vi "MainScan.vi"() -> ()   [LabVIEW 2012]
uses:
  <userlib>/Circular Buffer/Controls/Circular Buffer Operations.ctl
  <vilib>/DAQmx/write.llb/DAQmx Write (Digital Bool 1Line 1Point).vi
  <vilib>/DAQmx/write.llb/DAQmx Write (Analog 1D DBL NChan 1Samp).vi
  <vilib>/DAQmx/read.llb/DAQmx Read (Analog 1D DBL 1Chan NSamp).vi
  <vilib>/DAQmx/write.llb/DAQmx Write (Analog DBL 1Chan 1Samp).vi
  <vilib>/DAQmx/write.llb/DAQmx Write (Analog 2D DBL NChan NSamp).vi
  <vilib>/DAQmx/read.llb/DAQmx Read (Analog 1D Wfm NChan NSamp).vi
  <vilib>/DAQmx/create/channels.llb/DAQmx Create Channel (DO-Digital Output).vi
  <vilib>/DAQmx/create/channels.llb/DAQmx Create Channel (AO-Voltage-Basic).vi
  <vilib>/DAQmx/create/channels.llb/DAQmx Create Channel (AI-Voltage-Basic).vi
  <vilib>/DAQmx/configure/timing.llb/DAQmx Timing (Sample Clock).vi
  <vilib>/DAQmx/miscellaneous.llb/DAQmx Fill In Error Info.vi
  <vilib>/DAQmx/create/channels.llb/DAQmx Create Channel (CO-Pulse Generation-Frequency).vi
  <vilib>/DAQmx/configure/timing.llb/DAQmx Timing (Implicit).vi
  <vilib>/Analysis/baseanly.llb/Mean (DBL).vi
  <vilib>/DAQmx/configure/trigger.llb/DAQmx Start Trigger (Digital Edge).vi
  <userlib>/Circular Buffer/Instance VIs/Circular Buffer(2D Wfm).vi
  <vilib>/measure/madcrms.llb/Basic Averaged DC-RMS for N Chan.vi
  <resource>/objmgr/daqmx.rc
  <userlib>/Circular Buffer/Circular Buffer.lvlib
  <vilib>/Analysis/NI_AALBase.lvlib
  <vilib>/measure/NI_MAPro.lvlib
panel:
  in  "z-Position":dbl min=0.0 max=10.0
  in  "Schritte":dbl=20.0 min=0.0 step=1.0 format="%#.0f"
  out "Duration (m.s)":string
  in  "Piezo Stage":bool
  in  "maximum":dbl=1.0
  in  "minimum":dbl=-10.0
  out "Sensitivity":string
  out "Phase":string
  out "Lock-in":bool
  in  "green PMT-gain":dbl=5.0
  in  "red PMT-gain":dbl=9.5
  in  "NA 2":dbl=1.3 min=0.0
  in  "Magn":dbl=40.0
  in  "Magn":dbl=100.0
  in  "Buffer Size":i32(ring)=750 items=["1000x"=1000, "750x"=750, "500x"=500, "250x"=250, "150x"=150, "100x"=100, "50x"=50, "20x"=20]
  out "Buffer":dbl(slide) scale=0.0..1.0
  out "Mira Power (mW)":dbl format="%.2f"
  in  "Scanrate (pixels/s)":i32(ring)=50 items=["250 kHz"=250000, "200 kHz"=200000, "100 kHz"=100000, "50 kHz"=50000, "25 kHz"=25000, "20 kHz"=20000, "10 kHz"=10000, "5 kHz"=5000, "2 kHz"=2000, "1 kHz"=1000, "500 Hz"=500, "200 Hz"=200, "100 Hz"=100, "50 Hz"=50, "20 Hz"=20, "10 Hz"=10, "5 Hz"=5, "2 Hz"=2, "1 Hz"=1]
  out "Optimal":string
  out "Pixel [nm]":dbl format="%#.0f"
  in  "Pulse width fs":dbl=270.0 min=0.0
  in  "Power mW nosync":dbl=1.0 min=0.0
  in  "Power mW sync":dbl=1.0 min=0.0
  in  "Power mA":dbl=1.0 min=0.0
  in  "HWP":dbl=20.0 min=0.0 step=2.5
  in  "NA":dbl=1.2 min=0.0
  in  "Fire":bool
  in  "Pulse repetition rate":dbl(ring)=250000.0 items=["0.5 Hz"=0.5, "1 Hz"=1.0, "2 Hz"=2.0, "5 Hz"=5.0, "10 Hz"=10.0, "20 Hz"=20.0, "50 Hz"=50.0, "100 Hz"=100.0, "200 Hz"=200.0, "500 Hz"=500.0, "1 kHz"=1000.0, "2 kHz"=2000.0, "5 kHz"=5000.0, "10 kHz"=10000.0, "20 kHz"=20000.0, "50 kHz"=50000.0, "100 kHz"=100000.0, "200 kHz"=200000.0, "250 kHz"=250000.0]
  in  "Number of shots":i32(ring)=1 items=["Single"=1, "Double"=2, "5"=5, "10"=10, "20"=20, "50"=50, "100"=100, "200"=200, "500"=500, "1000"=1000, "2000"=2000, "5000"=5000, "10000"=10000, "20000"=20000, "50000"=50000, "100000"=100000, "200000"=200000, "500000"=500000, "Continuos"=0]
  in  "Swap Memory":bool
  out "Memory":dbl[][](graph)
  out "System":bool
  in  "black point":bool
  in  "Magnification":dbl=60.0
  in  "Go home":bool
  in  "Go to white point":bool
  in  "Maximum val":dbl max=100.0 format="%#_4f"
  in  "Minimum val":dbl min=-200.0 step=0.25 format="%#_4f"
  in  "Z-Stacking":bool
  in  "Schrittweite":dbl=1.0 min=0.0
  in  "Minimum":dbl(slide) min=-200.0 max=10.0 step=0.25 scale=-100.0..100.0
  in  "Maximum":dbl(slide)=0.30612244897959184 min=-10.0 max=100.0 scale=-100.0..100.0
  out "path":path
  in  "File identifier":string="unnamed_file"
  in  "Bild speichern ...":bool
  out "Grösse manuell":dbl=22.400000000000002
  in  "Scan":bool
  in  "y-Offset":dbl min=-636.16 max=636.16 format="%#.2f"
  in  "x-Offset":dbl min=-636.16 max=636.16 format="%#.2f"
  in  "Grösse":dbl(ring)=0.04 items=["1x1 µm"=0.005, "2x2 µm"=0.01, "4x4 µm"=0.02, "9x9 µm"=0.04, "18x18 µm"=0.08, "36x36 µm"=0.16, "72x72 µm"=0.32, "143x143 µm"=0.64]
  out "Image":dbl[][](graph)
  in  "Auflösung":i32(ring) items=["512x512"=512, "256x256"=256, "128x128"=128, "64x64"=64, "32x32"=32, "16x16"=16, "8x8"=8, "4x4"=4, "2x2"=2, "1x1"=1, "Optimal"=0]
  # "Auslesebereich"
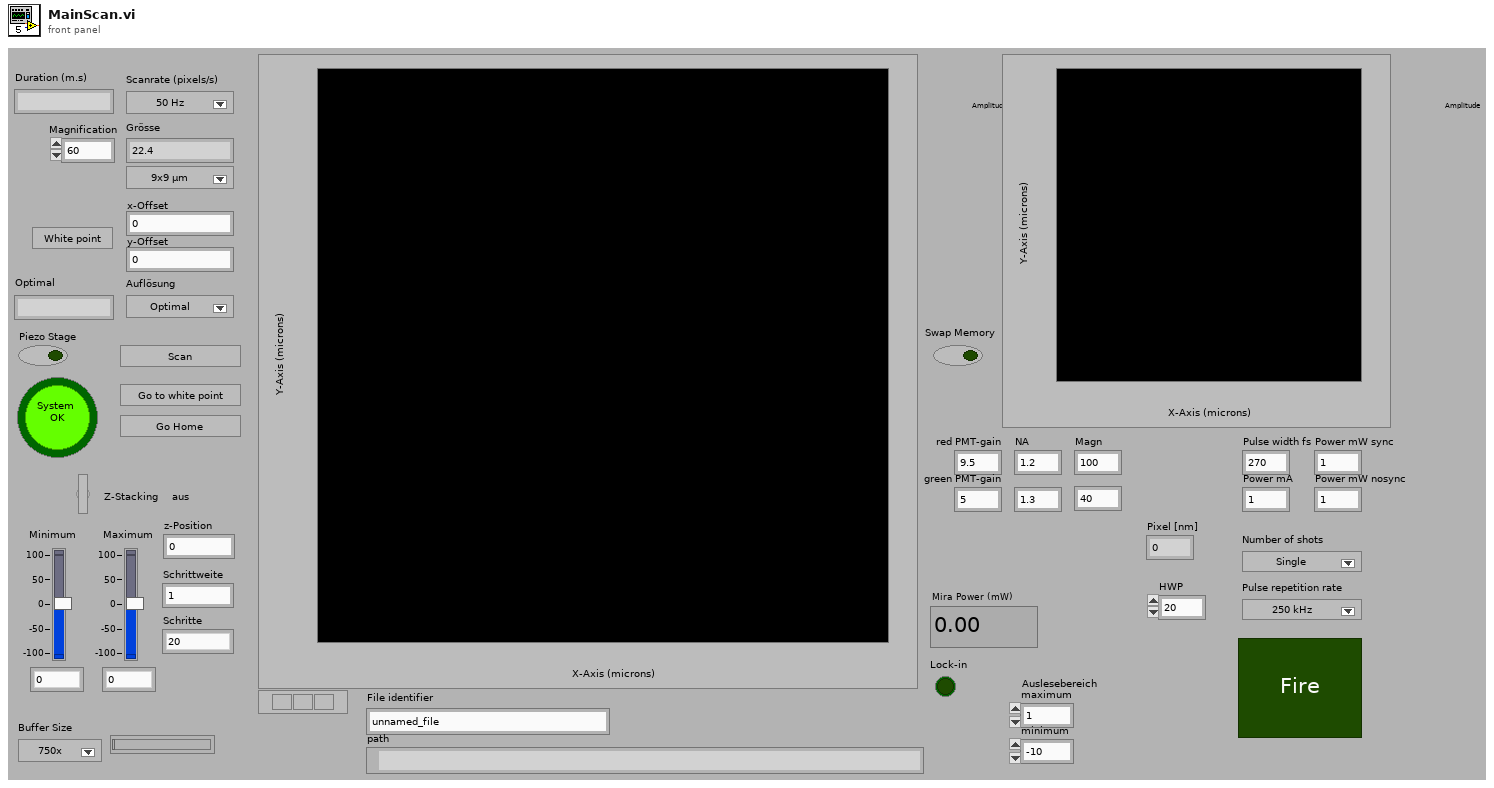
[diagram p1: front panel]
types:
  T1 = typedef "Circular Buffer.lvlib/Circular Buffer Operations.ctl" = enum16{"Initialize", "Get Backlog", "Write", "Read (continuous)", "Read (most recent)"}
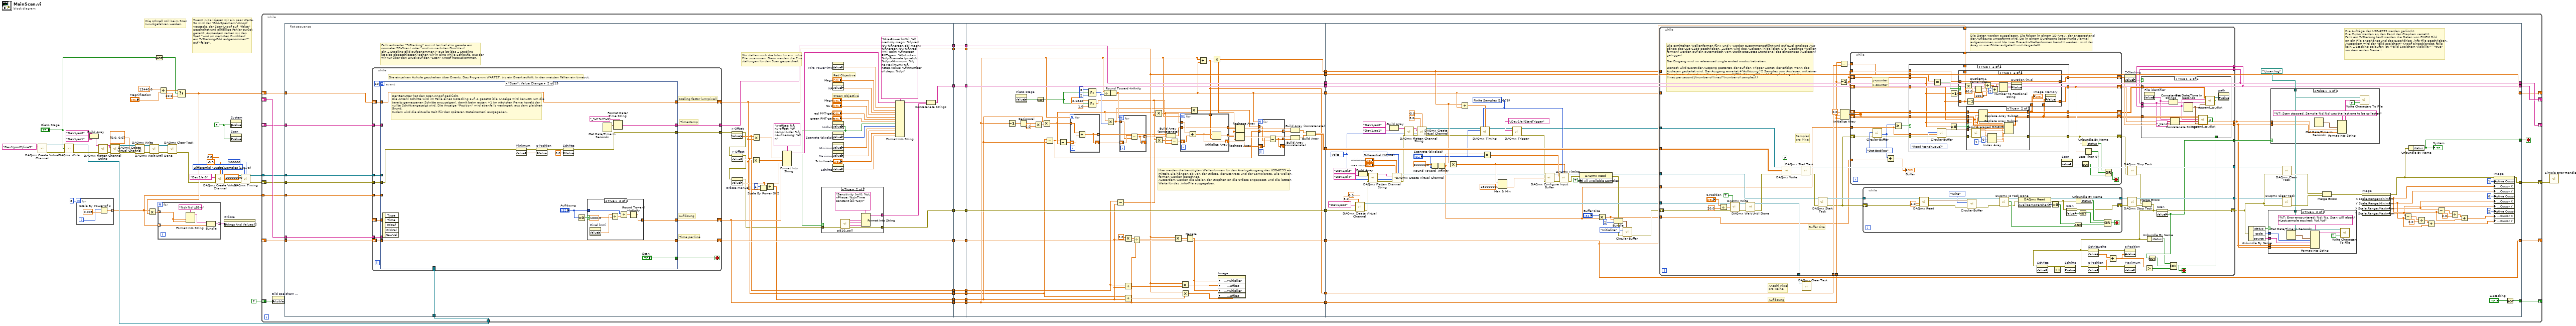
[diagram p0: block diagram]
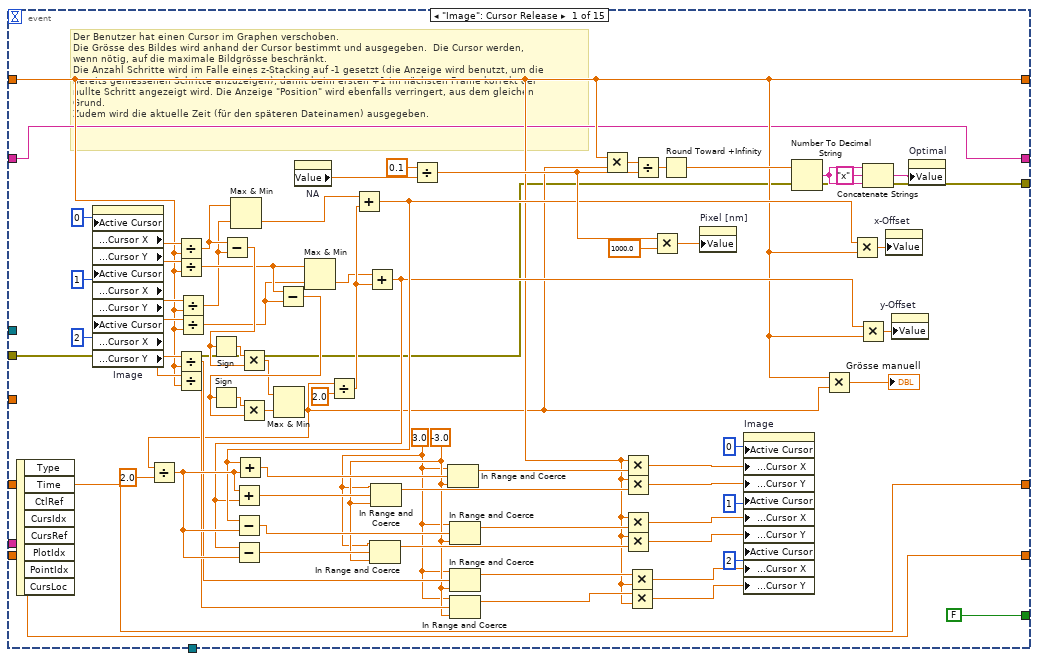
[diagram p2: hidden frame]
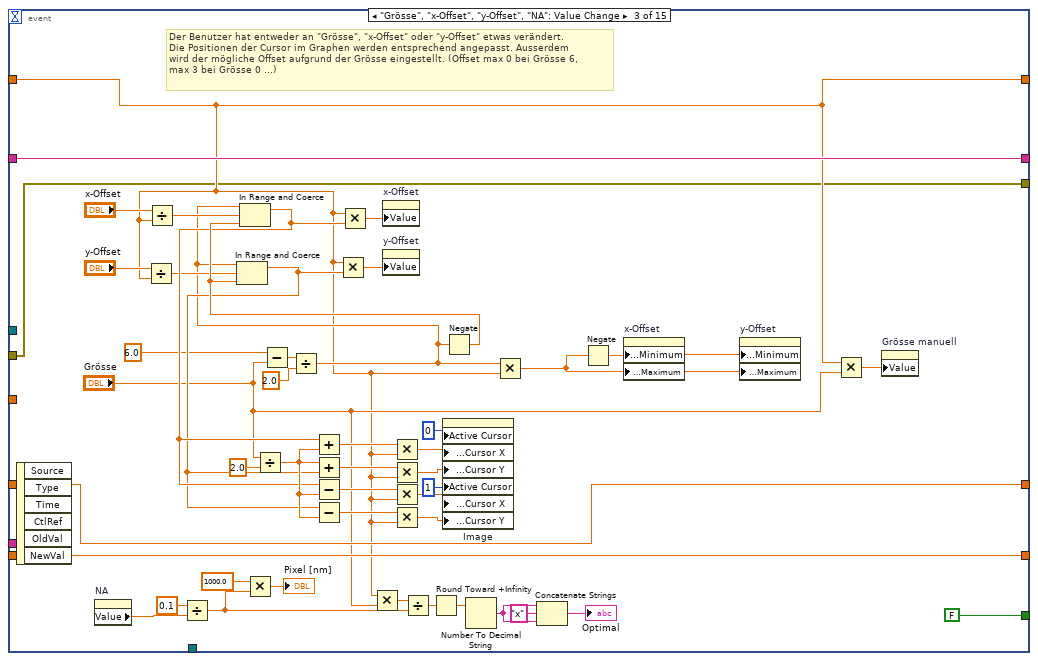
[diagram p4: hidden frame]
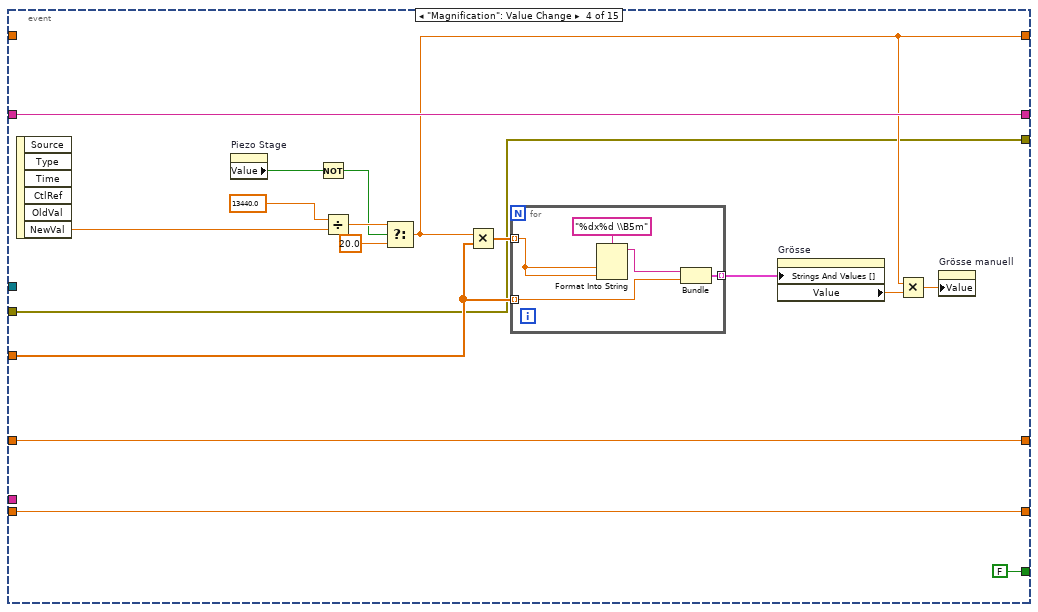
[diagram p5: hidden frame]
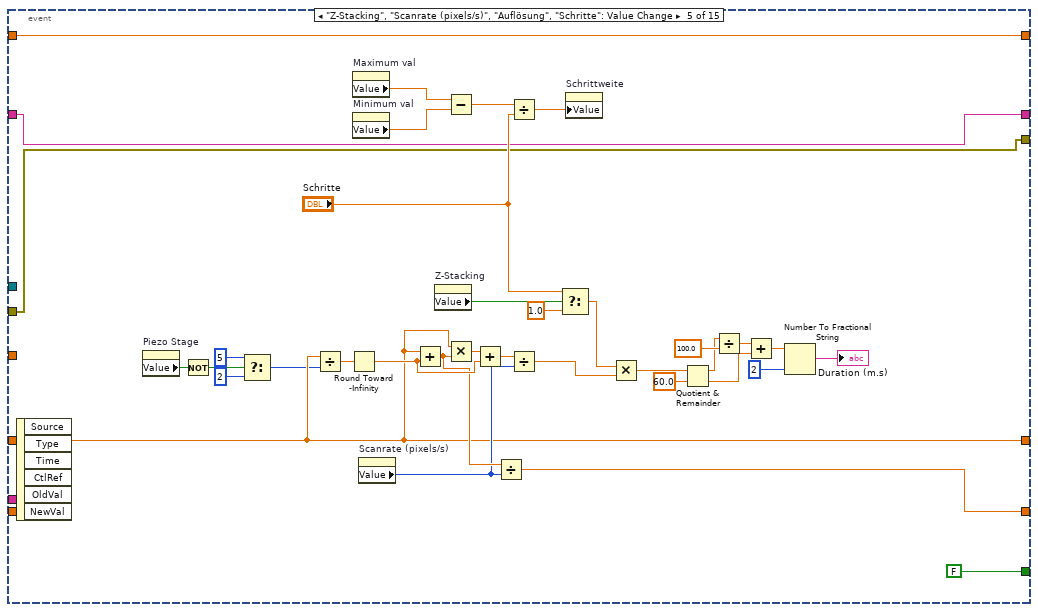
[diagram p6: hidden frame]
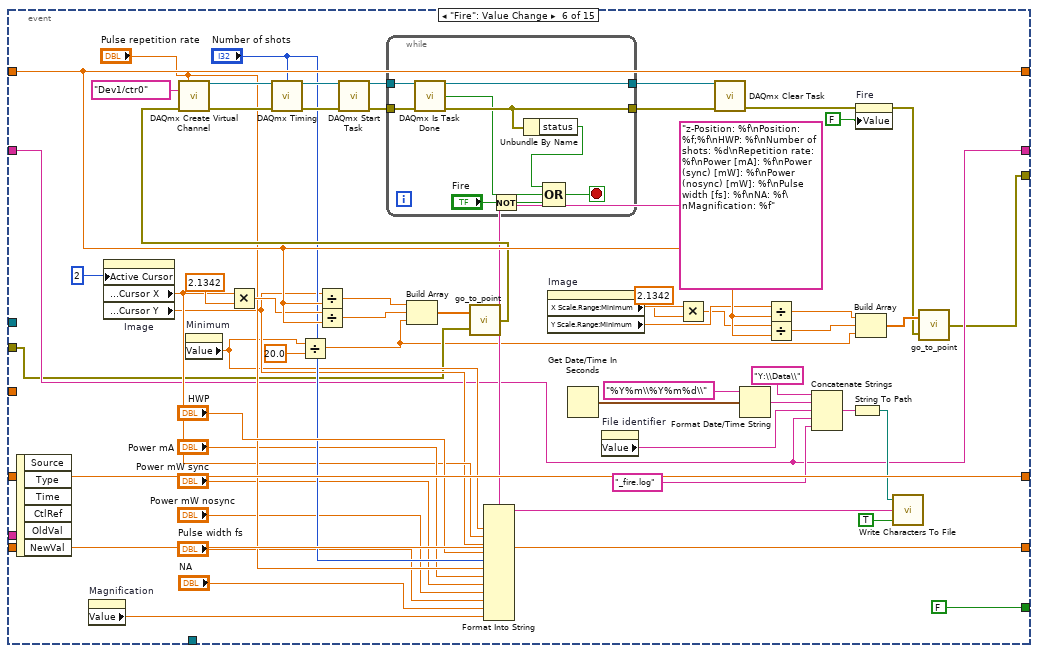
[diagram p7: hidden frame]
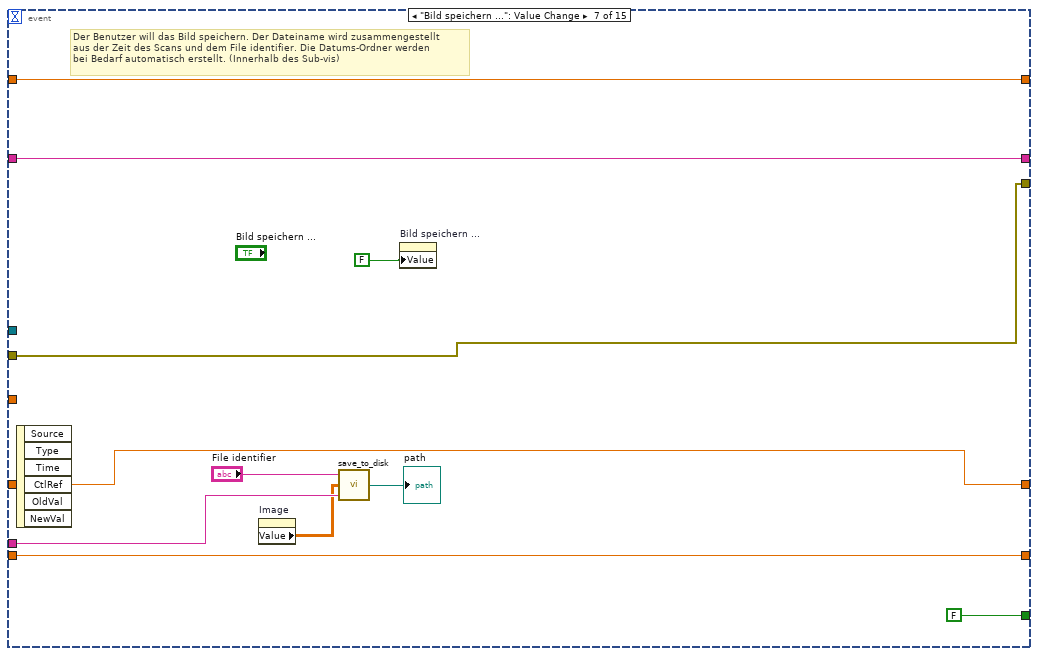
[diagram p8: hidden frame]
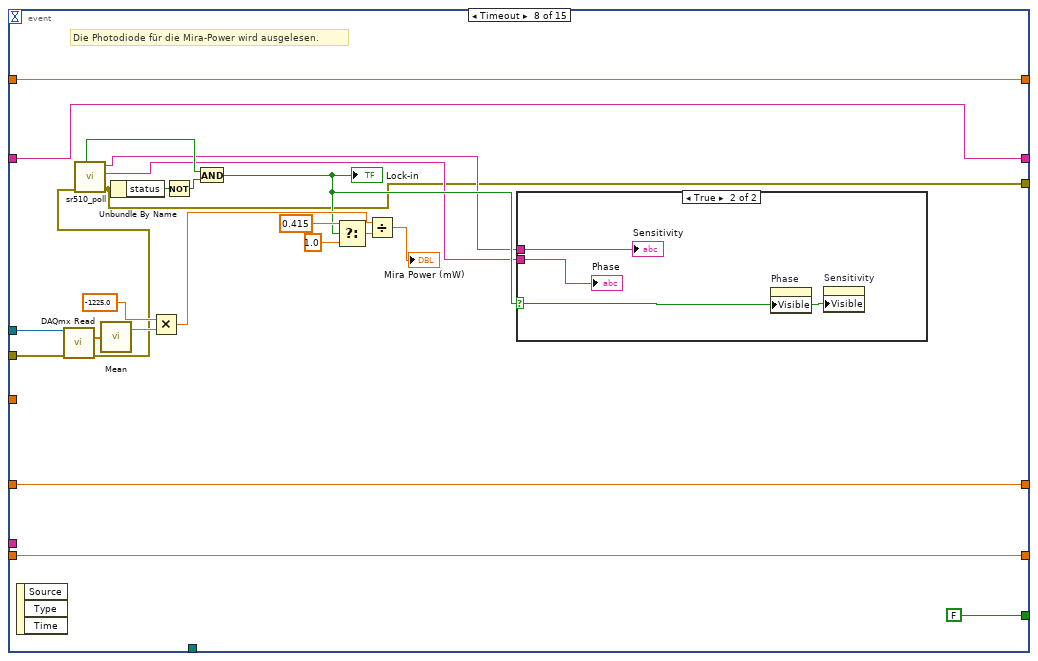
[diagram p9: hidden frame]
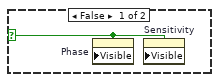
[diagram p10: hidden frame]
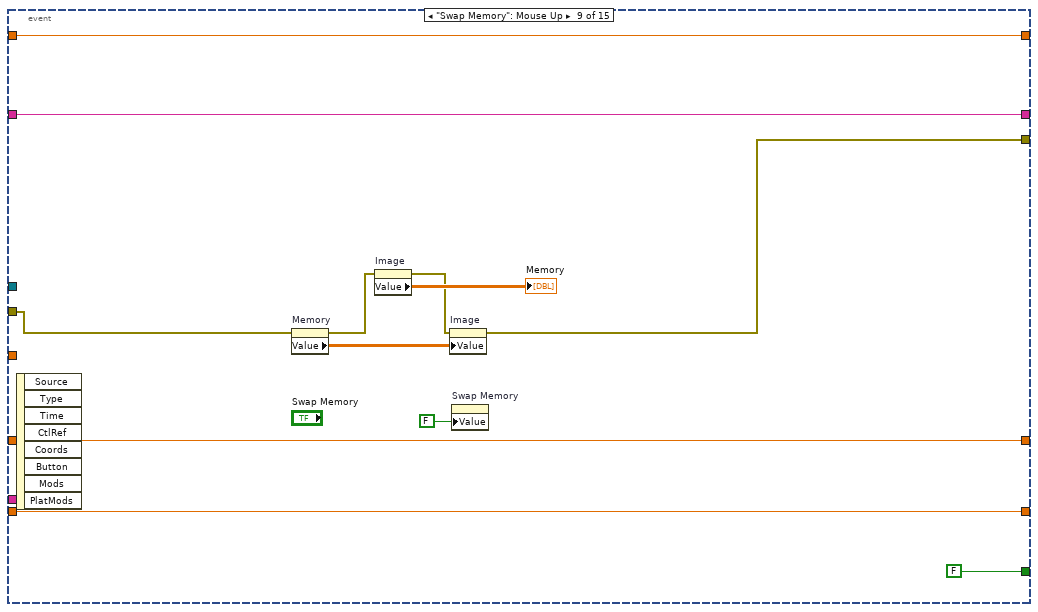
[diagram p11: hidden frame]
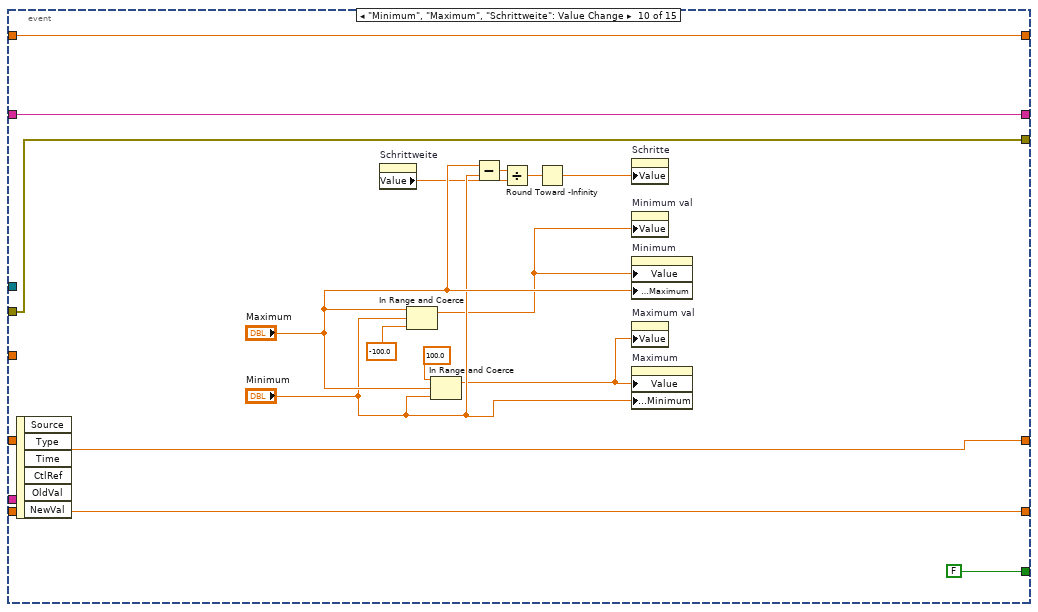
[diagram p12: hidden frame]
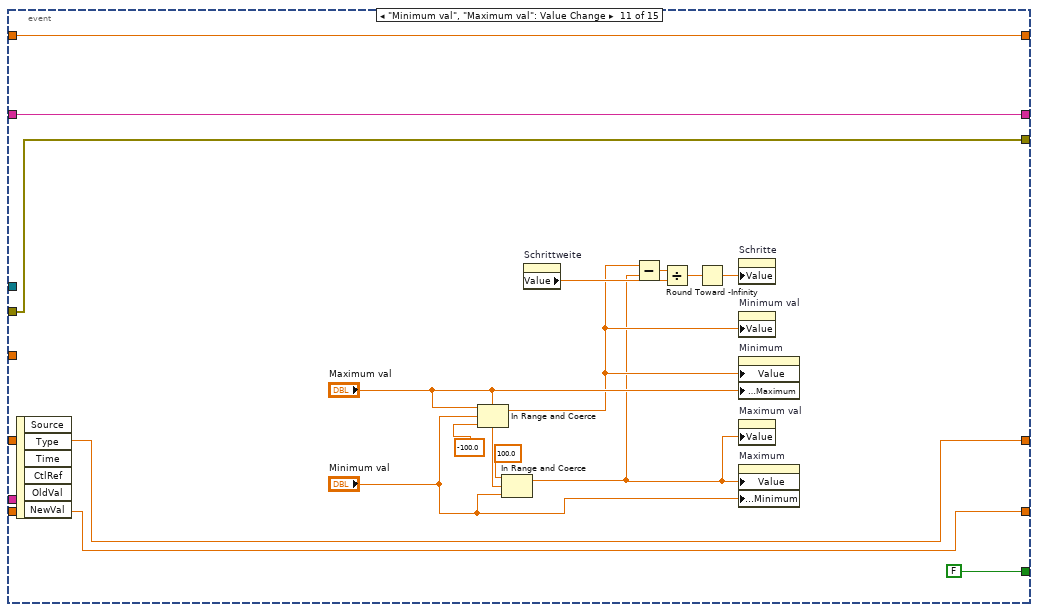
[diagram p13: hidden frame]
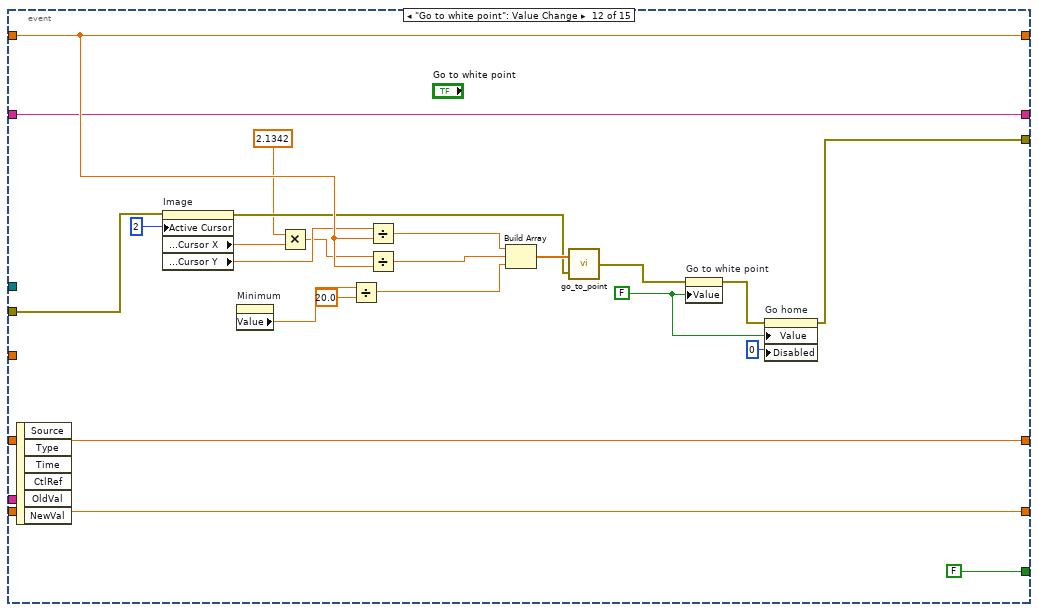
[diagram p14: hidden frame]
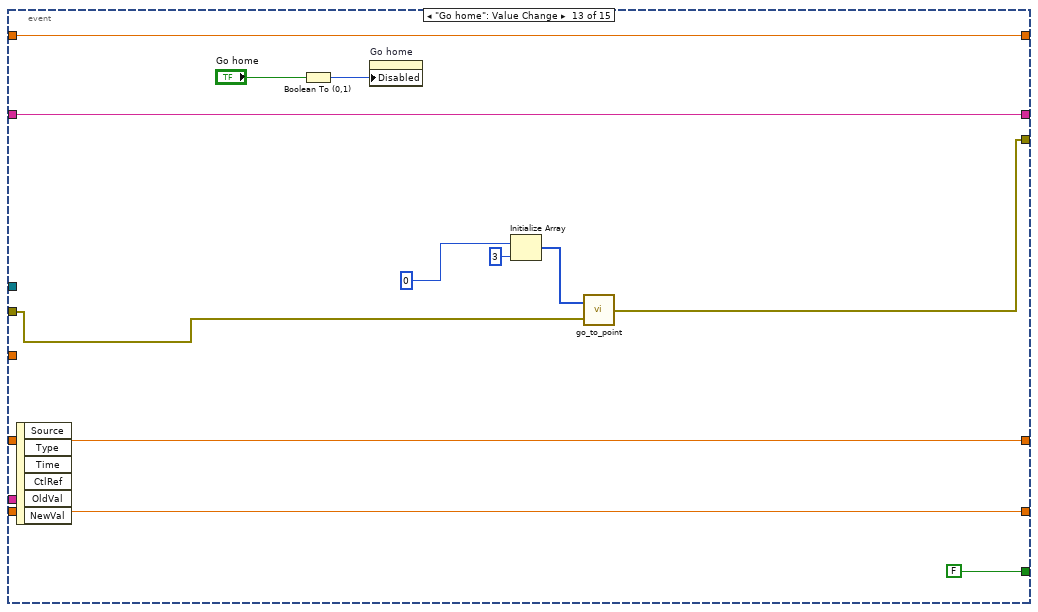
[diagram p15: hidden frame]
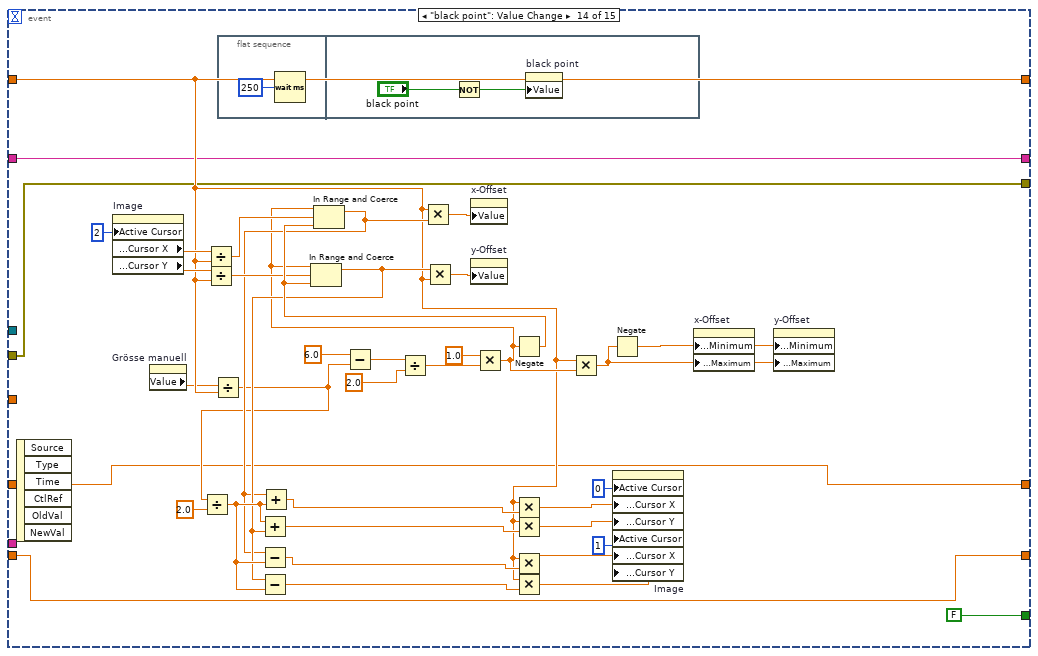
[diagram p16: hidden frame]
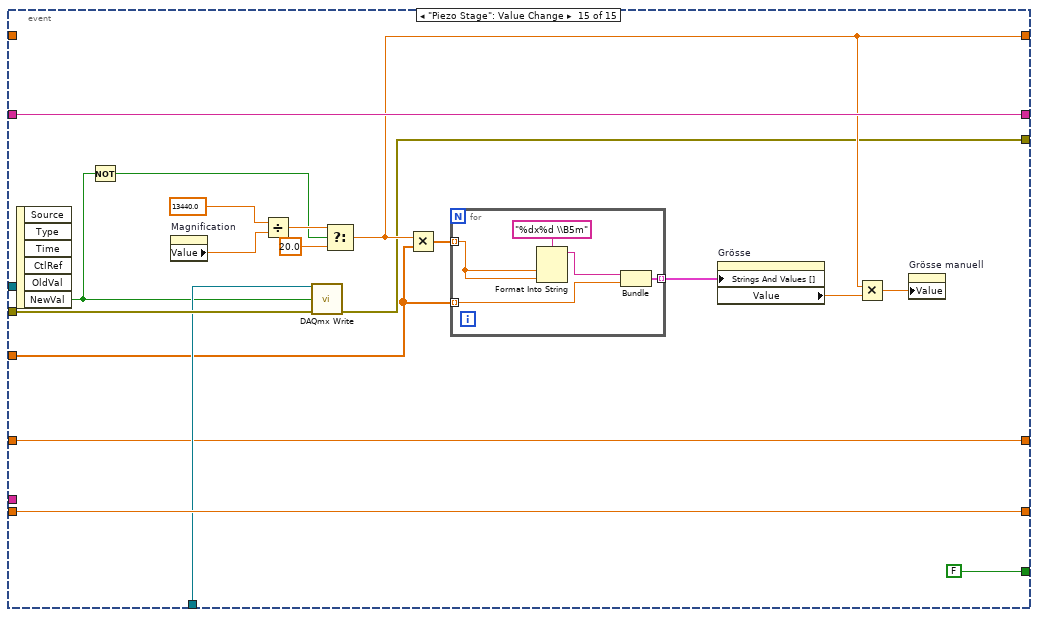
[diagram p17: hidden frame]
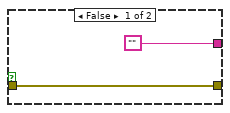
[diagram p18: hidden frame]
diagram:
  w15 = 10178 items=["Finite Samples"=10178, "Continuous Samples"=10123, "Hardware Timed Single Point"=12522] ("sample mode")
  w21 = 10106 items=["default"=-1, "RSE"=10083, "NRSE"=10078, "Differential"=10106, "Pseudodifferential"=12529] ("input terminal configuration")
  w1 = FALSE ("System")
  # "Wie schnell soll beim Scan\nzurückgefahren werden."
  # "Zuerst initialisieren wir ein paar Werte.\nSo wird der \"Bild-Speichern\"-Knopf\nversteckt, der Scan-Lnopf auf  \"false\"\ngeschaltet und allfällige Fehler zurück\ngesetzt. Ausserdem setzen wir den \nWert \"wird im nächsten Durchlauf\nein Z-Stacking-Bild aufgenommen?\"\nauf \"false\"."
  n1 = call-poly <vilib>:"DAQmx Create Virtual Channel.vi"("lines"=tag "Dev1/port2/line5") -> ("task out"=w26:refnum<k21>, "error out"=w25:errorcluster)  [unwired: 13 in]
  n2 = call-poly <vilib>:"DAQmx Write.vi"("task/channels in"=w26, "data"="Piezo Stage", "error in"=w25) -> ("task out"=w11:refnum<k21>, "error out"=w23:errorcluster)  [unwired: 10 in, 1 out]
  n3 = for {
    N: 8 -> [_]
    tunnel: [w45] -> w2 mode=indexing
    i -> [w44]
    n4 = Scale By Power Of 2(n=w44, x=0.005) -> (x*2^n=w45:dbl)
  }
  n5 = Build Array(tag "Dev1/ao0" ("physical channels"), tag "Dev1/ao1" ("physical channels")) -> (w38:tag[])
  n6 = call <vilib>:"DAQmx Flatten Channel String.vi"("names in"=w38, "error in"=w23) -> ("names out"=w37:string, "error out"=w36:errorcluster)  [unwired: 12 in]
  n7 = call-poly <vilib>:"DAQmx Create Virtual Channel.vi"("physical channels"=w37, "error in"=w36) -> ("task out"=w34:refnum<k21>, "error out"=w33:errorcluster)  [unwired: 12 in]
  n8 = call-poly <vilib>:"DAQmx Write.vi"("task/channels in"=w34, "data"=dbl[] [0.0, 0.0], "error in"=w33) -> ("task out"=w7:refnum<k21>, "error out"=w4:errorcluster)  [unwired: 10 in, 1 out]
  n9 = call <vilib>:"DAQmx Wait Until Done.vi"("task/channels in"=w7, "error in"=w4) -> ("task out"=w5:refnum<k21>, "error out"=w3:errorcluster)  [unwired: 12 in]
  n10 = Not(x="Piezo Stage") -> (.not. x?=w9:bool)
  n11 = Divide(x=13440.0, y="Magnification") -> (x/y=w31:dbl)
  n12 = call <vilib>:"DAQmx Clear Task.vi"("task in"=w5, "error in"=w3) -> ("error out"=w6:errorcluster)  [unwired: 13 in]
  n13 = Select(t=w31, s=w9, f=20.0) -> (s? t:f=w27:dbl)
  n14 = Multiply(x=w2, y=w27) -> (x*y=w28:dbl[])
  n15 = for {
    tunnel: w28 -> [w48] mode=indexing
    tunnel: [w51] -> w8 mode=indexing
    tunnel: w2 -> [w50] mode=indexing
    n16 = Format Into String(format string="%dx%d \\B5m", w48, w48) -> (resulting string=w47:string)  [unwired: 2 in, 1 out]
    n17 = Bundle(w47, w50) -> (w51:cluster{string, dbl})  [unwired: 1 in]
  }
  n18 = call-poly <vilib>:"DAQmx Create Virtual Channel.vi"("maximum value"=0.0, "minimum value"=-0.5, "input terminal configuration"=w21, "physical channels"=tag "Dev1/ai0", "error in"=w6) -> ("task out"=w17:refnum<k21>, "error out"=w18:errorcluster)  [unwired: 9 in]
  n19 = property on="Grösse" class="Ring (strict)"("Strings And Values []"=w8) -> ()  [unwired: 2 in, 2 out]
  n20 = property on="System" class="Bool (strict)"("Value"=w1) -> ()  [unwired: 2 in, 2 out]
  n21 = property on="Scan" class="Bool (strict)"("Value"=w1) -> ()  [unwired: 2 in, 2 out]
  n22 = call-poly <vilib>:"DAQmx Timing.vi"("task/channels in"=w17, "sample mode"=w15, "samples per channel"=100000, "rate"=1000000.0, "error in"=w18) -> ("task out"=w13:refnum<k21>, "error out"=w12:errorcluster)  [unwired: 9 in]
  n23 = while {
    shift-right: [w95] -> w40
    shift-left: w12 -> [w80]
    shift-right: [w89] -> _
    shift-left: FALSE ("Visible") -> [w94]
    shift-right: [w93] -> _
    shift-left: _ -> [w92]
    shift-right: [w91] -> _
    shift-left: _ -> [w90]
    tunnel: w2 -> [w88]
    shift-right: [w87] -> _
    shift-left: w27 -> [w86]
    tunnel: w13 -> [w84]
    shift-right: [w83] -> _
    shift-left: _ -> [w82]
    tunnel: w11 -> [w81]
    stop <- w85 stop-if-true
    n24 = property on="Bild speichern ..." class="Bool (strict)"("Visible"=w94) -> ()  [unwired: 2 in, 2 out]
    n25 = flat-sequence {
      tunnel: [w139] -> w69
      tunnel: [w113] -> w67
      tunnel: [w112] -> w65
      tunnel: [w109] -> w63
      tunnel: [w102] -> w61
      tunnel: [w101] -> w59
      tunnel: [w138] -> w57
      tunnel: [w110] -> w55
      tunnel: [w137] -> w53
      tunnel: w81 -> [w130]
      tunnel: w82 -> [w131]
      tunnel: w84 -> [w132]
      tunnel: w80 -> [w133]
      tunnel: w86 -> [w134]
      tunnel: w88 -> [w135]
      tunnel: w90 -> [w115]
      tunnel: w92 -> [w136]
      tunnel: w69 -> [w618]
      tunnel: [w618] -> w68
      tunnel: w67 -> [w617]
      tunnel: [w617] -> w66
      tunnel: w65 -> [w616]
      tunnel: [w616] -> w64
      tunnel: w63 -> [w615]
      tunnel: [w615] -> w62
      tunnel: w61 -> [w614]
      tunnel: [w614] -> w60
      tunnel: w59 -> [w613]
      tunnel: [w613] -> w58
      tunnel: w57 -> [w612]
      tunnel: [w612] -> w56
      tunnel: w55 -> [w611]
      tunnel: [w611] -> w54
      tunnel: w53 -> [w610]
      tunnel: [w610] -> w52
      tunnel: [w657] -> w70
      tunnel: w68 -> [w657]
      tunnel: w66 -> [w626]
      tunnel: w64 -> [w627]
      tunnel: w62 -> [w658]
      tunnel: w60 -> [w668]
      tunnel: w58 -> [w669]
      tunnel: [w669] -> w71
      tunnel: [w673] -> w72
      tunnel: w56 -> [w673]
      tunnel: w54 -> [w667]
      tunnel: [w667] -> w73
      tunnel: [w668] -> w74
      tunnel: [w647] -> w75
      tunnel: [w655] -> w76
      tunnel: [w646] -> w77
      tunnel: [w645] -> w78
      tunnel: [w621] -> w79
      tunnel: w52 -> [w621]
      tunnel: [w758] -> w95
      tunnel: [w695] -> w93
      tunnel: [w696] -> w91
      tunnel: [w697] -> w89
      tunnel: [w699] -> w87
      tunnel: [w771] -> w85
      tunnel: [w770] -> w83
      tunnel: w70 -> [w769]
      tunnel: w71 -> [w695]
      tunnel: w72 -> [w696]
      tunnel: w73 -> [w699]
      tunnel: w74 -> [w753]
      tunnel: w75 -> [w757]
      tunnel: w76 -> [w720]
      tunnel: w77 -> [w768]
      tunnel: w78 -> [w719]
      tunnel: w79 -> [w770]
      frame #0 {
        # "Falls entweder \"Z-Stacking\" aus ist (es lief also gerade ein\nnormaler 2D-Scan), oder \"wird im nächsten Durchlauf\nein Z-Stacking-Bild aufgenommen?\" aus ist (das Z-Stacking\nist also abgeschlossen) gehen wir in eine while-Schlaufe, aus der\nwir nur über den Druck auf den \"Scan\"-Knopf herauskommen."
        # "Red Objective"
        # "Green Objective"
        # "Wir stellen noch die Infos für ein .info-\nFile zusammen. Darin werden die Ein-\nstellungen für den Scan gespeichert."
        n26 = while {
          tunnel: w136 -> [w154]
          tunnel: w135 -> [w153]
          shift-right: [w151] -> w110
          shift-left: w134 -> [w152]
          tunnel: w132 -> [w149]
          tunnel: w133 -> [w148]
          shift-right: [w147] -> w137
          shift-left: w131 -> [w146]
          tunnel: w130 -> [w145]
          shift-right: [w143] -> w139
          shift-left: _ -> [w142]
          tunnel: w115 -> [w150]
          tunnel: [w141] -> w138
          tunnel: [w140] -> w104
          stop <- w144 stop-if-true
          # "Time per line"
          # "Timestamp"
          # "Auflösung"
          # "Scaling factor (um/pixel)"
          # "Die einzelnen Aufrufe geschehen über Events. Das Programm WARTET, bis ein Event auftritt. In den meisten Fällen ein timeout."
          n27 = event shown="[1] \"Scan\": Value Change" {
            selector: _ -> [_ _ _ _ _ _ _ _ _ _ _ _ _ _ _]
            dyn-events: _ -> [_ _ _ _ _ _ _ _ _ _ _ _ _ _ _]
            timeout: 10 -> [_ _ _ _ _ _ _ _ _ _ _ _ _ _ _]
            tunnel: w154 -> [_ _ _ _ _ _ w426 _ _ _ _ _ _ _ _]
            tunnel: w153 -> [_ _ _ w306 _ _ _ _ _ _ _ _ _ _ w583]
            tunnel: [w160 w233 w250 w296 w324 w409 w425 w452 w466 w475 w494 w521 w533 w543 w579] -> w151
            tunnel: w152 -> [w160 w233 w250 _ w324 w409 w425 w452 w466 w475 w494 w521 w533 w543 _]
            tunnel: w150 -> [w157 _ w253 w302 w323 w359 w420 w431 w459 w471 w487 w506 w529 w537 w590]
            tunnel: w149 -> [_ _ _ _ _ _ _ w451 _ _ _ _ _ _ _]
            tunnel: w148 -> [w156 w230 w249 w295 w317 w358 w419 w450 w458 w469 w485 w505 w528 w536 w594]
            tunnel: [w167 w240 w256 w299 w334 w408 w424 w432 w465 w474 w490 w517 w532 w540 w595] -> w147
            tunnel: w146 -> [w167 w240 w256 w299 _ w408 w424 w432 w465 w474 w490 w517 w532 w540 w595]
            tunnel: w145 -> [_ _ _ _ _ _ _ _ _ _ _ _ _ _ w593]
            tunnel: [FALSE ("Scan") "Scan" FALSE ("Scan") FALSE ("Scan") FALSE ("Scan") FALSE ("Scan") FALSE ("Scan") FALSE ("Scan") FALSE ("Scan") FALSE ("Scan") FALSE ("Scan") FALSE ("Scan") FALSE ("Scan") FALSE ("Scan") FALSE ("Scan")] -> w144
            tunnel: [w158 w237 w254 w300 w332 w406 w421 w433 w460 w472 w488 w508 w530 w538 w591] -> w143
            tunnel: w142 -> [w158 _ w254 w300 w332 w406 w421 w433 w460 w472 w488 w508 w530 w538 w591]
            tunnel: [w157 w236 w253 w302 w323 w359 w420 w431 w459 w471 w487 w506 w529 w537 w590] -> w141
            tunnel: [w156 w227 w249 w295 w317 w357 w419 w430 w457 w469 w485 w504 w527 w536 w578] -> w140
            event "Image": Cursor Release {
              w179 = 3.0 ("upper limit")
              w180 = -3.0 ("upper limit")
              # "Der Benutzer hat einen Cursor im Graphen verschoben.\nDie Grösse des Bildes wird anhand der Cursor bestimmt und ausgegeben.  Die Cursor werden, \nwenn nötig, auf die maximale Bildgrösse beschränkt.\nDie Anzahl Schritte wird im Falle eines z-Stacking auf -1 gesetzt (die Anzeige wird benutzt, um die \nbereits gemessenen Schritte anzuzeigen), damit beim ersten +1 im nächsten Frame korrekt der \nnullte Schritt angezeigt wird. Die Anzeige \"Position\" wird ebenfalls verringert, aus dem gleichen \nGrund.\nZudem wird die aktuelle Zeit (für den späteren Dateinamen) ausgegeben."
              n28 = event-data() -> ()  [unwired: 1 in, 8 out]
              n29 = property on="Image" class="IntGraph (strict)"("Active Cursor"=u32 0, "Active Cursor"=u32 1, "Active Cursor"=u32 2) -> ("Cursor.Cursor Position:Cursor X"=w198:dbl, "Cursor.Cursor Position:Cursor Y"=w197:dbl, "Cursor.Cursor Position:Cursor X"=w196:dbl, "Cursor.Cursor Position:Cursor Y"=w195:dbl, "Cursor.Cursor Position:Cursor X"=w189:dbl, "Cursor.Cursor Position:Cursor Y"=w188:dbl)  [unwired: 2 in, 2 out]
              n30 = Divide(x=w198, y=w160) -> (x/y=w194:dbl)
              n31 = Divide(x=w197, y=w160) -> (x/y=w193:dbl)
              n32 = Divide(x=w189, y=w160) -> (x/y=w182:dbl)
              n33 = Divide(x=w188, y=w160) -> (x/y=w181:dbl)
              n34 = Divide(x=w196, y=w160) -> (x/y=w192:dbl)
              n35 = Divide(x=w195, y=w160) -> (x/y=w191:dbl)
              n36 = Subtract(x=w194, y=w192) -> (x-y=w223:dbl)
              n37 = Sign(1:w223) -> (0:w224:dbl)
              n38 = Max & Min(x=w194, y=w192) -> (min(x,y)=w216:dbl)  [unwired: 1 out]
              n39 = Multiply(x=w224, y=w223) -> (x*y=w218:dbl)
              n40 = Subtract(x=w193, y=w191) -> (x-y=w221:dbl)
              n41 = Sign(1:w221) -> (0:w222:dbl)
              n42 = Multiply(x=w222, y=w221) -> (x*y=w217:dbl)
              n43 = Max & Min(x=w218, y=w217) -> (min(x,y)=w159:dbl)  [unwired: 1 out]
              n44 = Divide(x=w159, y=2.0) -> (x/y=w211:dbl)
              n45 = property on="NA" class="DigNum (strict)"() -> ("Value"=w172:dbl)  [unwired: 2 in, 2 out]
              n46 = Max & Min(x=w193, y=w191) -> (min(x,y)=w215:dbl)  [unwired: 1 out]
              n47 = Divide(x=w159, y=2.0) -> (x/y=w219:dbl)
              n48 = Add(x=w216, y=w219) -> (x+y=w164:dbl)
              n49 = Subtract(x=w164, y=w211) -> (x-y=w208:dbl)
              n50 = Add(x=w164, y=w211) -> (x+y=w210:dbl)
              n51 = Add(x=w215, y=w219) -> (x+y=w162:dbl)
              n52 = Add(x=w211, y=w162) -> (x+y=w209:dbl)
              n53 = Subtract(x=w162, y=w211) -> (x-y=w207:dbl)
              n54 = In Range and Coerce(upper limit=w179, x=w207, lower limit=w180) -> (coerced(x)=w206:dbl)  [unwired: 1 out]
              n55 = In Range and Coerce(upper limit=w179, x=w209, lower limit=w180) -> (coerced(x)=w204:dbl)  [unwired: 1 out]
              n56 = Divide(x=0.1, y=w172) -> (x/y=w170:dbl)
              n57 = In Range and Coerce(upper limit=w179, x=w210, lower limit=w180) -> (coerced(x)=w203:dbl)  [unwired: 1 out]
              n58 = In Range and Coerce(upper limit=w179, x=w208, lower limit=w180) -> (coerced(x)=w205:dbl)  [unwired: 1 out]
              n59 = In Range and Coerce(upper limit=w179, x=w182, lower limit=w180) -> (coerced(x)=w184:dbl)  [unwired: 1 out]
              n60 = In Range and Coerce(upper limit=w179, x=w181, lower limit=w180) -> (coerced(x)=w183:dbl)  [unwired: 1 out]
              n61 = Multiply(x=w160, y=w159) -> (x*y=w177:dbl)
              n62 = Multiply(x=w160, y=w203) -> (x*y=w199:dbl)
              n63 = Multiply(x=w160, y=w204) -> (x*y=w200:dbl)
              n64 = Multiply(x=w160, y=w205) -> (x*y=w201:dbl)
              n65 = Multiply(x=w160, y=w206) -> (x*y=w202:dbl)
              n66 = Multiply(x=w184, y=w160) -> (x*y=w186:dbl)
              n67 = Multiply(x=w183, y=w160) -> (x*y=w185:dbl)
              n68 = Divide(x=w177, y=w170) -> (x/y=w176:dbl)
              n69 = Multiply(x=w170, y=1000.0) -> (x*y=w169:dbl)
              n70 = Round Toward +Infinity(x=w176) -> (ceil(x): smallest int >= x=w175:dbl)
              n71 = property on="Pixel [nm]" class="DigNum (strict)"("Value"=w169) -> ()  [unwired: 2 in, 2 out]
              n72 = property on="Image" class="IntGraph (strict)"("Active Cursor"=u32 0, "Cursor.Cursor Position:Cursor X"=w199, "Cursor.Cursor Position:Cursor Y"=w200, "Active Cursor"=u32 1, "Cursor.Cursor Position:Cursor X"=w201, "Cursor.Cursor Position:Cursor Y"=w202, "Active Cursor"=u32 2, "Cursor.Cursor Position:Cursor X"=w186, "Cursor.Cursor Position:Cursor Y"=w185) -> ()  [unwired: 2 in, 2 out]
              n73 = Number To Decimal String(number=w175) -> (decimal integer string=w173:string)  [unwired: 1 in]
              n74 = Multiply(x=w160, y=w159) -> (x*y=→"Grösse manuell":dbl)
              n75 = Multiply(x=w164, y=w160) -> (x*y=w165:dbl)
              n76 = Multiply(x=w162, y=w160) -> (x*y=w163:dbl)
              n77 = Concatenate Strings(w173, "x" ("string"), w173) -> (w171:string)
              n78 = property on="x-Offset" class="DigNum (strict)"("Value"=w165) -> ()  [unwired: 2 in, 2 out]
              n79 = property on="y-Offset" class="DigNum (strict)"("Value"=w163) -> ()  [unwired: 2 in, 2 out]
              n80 = property on="Optimal" class="Str"("Value"=w171) -> ()  [unwired: 2 in, 2 out]
            }
            event "Scan": Value Change {
              # "Der Benutzer hat den Scan-Knopf gedrückt.\nDie Anzahl Schritte wird im Falle eines z-Stacking auf -1 gesetzt (die Anzeige wird benutzt, um die \nbereits gemessenen Schritte anzuzeigen), damit beim ersten +1 im nächsten Frame korrekt der \nnullte Schritt angezeigt wird. Die Anzeige \"Position\" wird ebenfalls verringert, aus dem gleichen \nGrund.\nZudem wird die aktuelle Zeit (für den späteren Dateinamen) ausgegeben."
              n81 = event-data() -> ()  [unwired: 1 in, 5 out]
              n82 = property on="Minimum" class="Slide (strict)"(error in=w230) -> (error out=w229:errorcluster, "Value"=w231:dbl)  [unwired: 1 in, 1 out]
              n83 = property on="z-Position" class="DigNum (strict)"(error in=w229, "Value"=w231) -> (error out=w228:errorcluster)  [unwired: 1 in, 1 out]
              n84 = property on="Schritte" class="DigNum (strict)"(error in=w228, "Value"=0.0 ("Schritte")) -> (error out=w227:errorcluster)  [unwired: 1 in, 1 out]
              n85 = Equal To 0?(x="Auflösung") -> (x = 0?=w238:bool)
              n86 = case shown="True" w238 {
                tunnel: "Auflösung" -> [w242 w243]
                tunnel: [w242 w247] -> w237
                frame False {
                }
                frame True {
                  n87 = property on="Pixel [nm]" class="DigNum (strict)"() -> ("Value"=w246:dbl)  [unwired: 2 in, 2 out]
                  n88 = Divide(x=w246, y=1000.0) -> (x/y=w245:dbl)
                  n89 = Divide(x=w243, y=w245) -> (x/y=w248:dbl)
                  n90 = Round Toward +Infinity(x=w248) -> (ceil(x): smallest int >= x=w247:dbl)
                }
              }
              n91 = Get Date/Time In Seconds() -> (seconds since 1Jan1904=w234:timestamp)
              n92 = Format Date/Time String(time format string (%c)="_%H%M%S", seconds (now)=w234) -> (date/time string=w236:string)  [unwired: 1 in]
            }
            event "Grösse", "x-Offset", "y-Offset", "NA": Value Change {
              # "Der Benutzer hat entweder an \"Grösse\", \"x-Offset\" oder \"y-Offset\" etwas verändert.\nDie Positionen der Cursor im Graphen werden entsprechend angepasst. Ausserdem\nwird der mögliche Offset aufgrund der Grösse eingestellt. (Offset max 0 bei Grösse 6,\nmax 3 bei Grösse 0 ...)"
              n93 = event-data() -> ()  [unwired: 1 in, 6 out]
              n94 = property on="NA" class="DigNum (strict)"() -> ("Value"=w267:dbl)  [unwired: 2 in, 2 out]
              n95 = Divide(x="y-Offset", y=w250) -> (x/y=w283:dbl)
              n96 = Divide(x="x-Offset", y=w250) -> (x/y=w286:dbl)
              n97 = Divide(x=0.1, y=w267) -> (x/y=w258:dbl)
              n98 = Multiply(x=1000.0, y=w258) -> (x*y=→"Pixel [nm]":dbl)
              n99 = Divide(x="Grösse", y=2.0) -> (x/y=w294:dbl)
              n100 = Subtract(x=6.0, y="Grösse") -> (x-y=w289:dbl)
              n101 = Divide(x=w289, y=2.0) -> (x/y=w279:dbl)
              n102 = Multiply(x=w250, y="Grösse") -> (x*y=w265:dbl)
              n103 = Divide(x=w265, y=w258) -> (x/y=w264:dbl)
              n104 = Round Toward +Infinity(x=w264) -> (ceil(x): smallest int >= x=w263:dbl)
              n105 = Negate(x=w279) -> (-x=w288:dbl)
              n106 = In Range and Coerce(upper limit=w279, x=w283, lower limit=w288) -> (coerced(x)=w280:dbl)  [unwired: 1 out]
              n107 = In Range and Coerce(upper limit=w279, x=w286, lower limit=w288) -> (coerced(x)=w285:dbl)  [unwired: 1 out]
              n108 = Add(x=w285, y=w294) -> (x+y=w272:dbl)
              n109 = Add(x=w294, y=w280) -> (x+y=w273:dbl)
              n110 = Subtract(x=w285, y=w294) -> (x-y=w274:dbl)
              n111 = Subtract(x=w280, y=w294) -> (x-y=w275:dbl)
              n112 = Multiply(x=w250, y=w280) -> (x*y=w281:dbl)
              n113 = Multiply(x=w250, y=w285) -> (x*y=w284:dbl)
              n114 = property on="x-Offset" class="DigNum (strict)"("Value"=w284) -> ()  [unwired: 2 in, 2 out]
              n115 = property on="y-Offset" class="DigNum (strict)"("Value"=w281) -> ()  [unwired: 2 in, 2 out]
              n116 = Multiply(x=w272, y=w250) -> (x*y=w268:dbl)
              n117 = Multiply(x=w273, y=w250) -> (x*y=w271:dbl)
              n118 = Multiply(x=w274, y=w250) -> (x*y=w270:dbl)
              n119 = Multiply(x=w275, y=w250) -> (x*y=w269:dbl)
              n120 = property on="Image" class="IntGraph (strict)"("Active Cursor"=u32 0, "Cursor.Cursor Position:Cursor X"=w268, "Cursor.Cursor Position:Cursor Y"=w271, "Active Cursor"=u32 1, "Cursor.Cursor Position:Cursor X"=w270, "Cursor.Cursor Position:Cursor Y"=w269) -> ()  [unwired: 2 in, 2 out]
              n121 = Number To Decimal String(number=w263) -> (decimal integer string=w261:string)  [unwired: 1 in]
              n122 = Multiply(x=w279, y=w250) -> (x*y=w278:dbl)
              n123 = Concatenate Strings(w261, "x" ("string"), w261) -> (→"Optimal":string)
              n124 = Negate(x=w278) -> (-x=w277:dbl)
              n125 = property on="x-Offset" class="DigNum (strict)"("Data Range:Minimum"=w277, "Data Range:Maximum"=w278) -> ()  [unwired: 2 in, 2 out]
              n126 = property on="y-Offset" class="DigNum (strict)"("Data Range:Minimum"=w277, "Data Range:Maximum"=w278) -> ()  [unwired: 2 in, 2 out]
              n127 = Multiply(x=w250, y="Grösse") -> (x*y=w252:dbl)
              n128 = property on="Grösse manuell" class="DigNum (strict)"("Value"=w252) -> ()  [unwired: 2 in, 2 out]
            }
            event "Magnification": Value Change {
              n129 = event-data() -> ("NewVal"=w303:dbl)  [unwired: 1 in, 5 out]
              n130 = property on="Piezo Stage" class="Bool (strict)"() -> ("Value"=w308:bool)  [unwired: 2 in, 2 out]
              n131 = Not(x=w308) -> (.not. x?=w307:bool)
              n132 = Divide(x=13440.0, y=w303) -> (x/y=w310:dbl)
              n133 = Select(t=w310, s=w307, f=20.0) -> (s? t:f=w296:dbl)
              n134 = Multiply(x=w296, y=w306) -> (x*y=w305:dbl[])
              n135 = for {
                tunnel: w305 -> [w312] mode=indexing
                tunnel: [w316] -> w304 mode=indexing
                tunnel: w306 -> [w315] mode=indexing
                n136 = Format Into String(format string="%dx%d \\B5m", w312, w312) -> (resulting string=w313:string)  [unwired: 2 in, 1 out]
                n137 = Bundle(w313, w315) -> (w316:cluster{string, dbl})  [unwired: 1 in]
              }
              n138 = property on="Grösse" class="Ring (strict)"("Strings And Values []"=w304) -> ("Value"=w298:dbl)  [unwired: 2 in, 2 out]
              n139 = Multiply(x=w296, y=w298) -> (x*y=w297:dbl)
              n140 = property on="Grösse manuell" class="DigNum (strict)"("Value"=w297) -> ()  [unwired: 2 in, 2 out]
            }
            event "Z-Stacking", "Scanrate (pixels/s)", "Auflösung", "Schritte": Value Change {
              n141 = event-data() -> ()  [unwired: 1 in, 6 out]
              n142 = property on="Piezo Stage" class="Bool (strict)"() -> ("Value"=w319:bool)  [unwired: 2 in, 2 out]
              n143 = Not(x=w319) -> (.not. x?=w318:bool)
              n144 = Select(t=u8 5, s=w318, f=u8 2) -> (s? t:f=w320:u8)
              n145 = Divide(x=w332, y=w320) -> (x/y=w351:dbl)
              n146 = Round Toward -Infinity(1:w351) -> (0:w349:dbl)
              n147 = property on="Maximum val" class="DigNum (strict)"() -> ("Value"=w331:dbl)  [unwired: 2 in, 2 out]
              n148 = property on="Minimum val" class="DigNum (strict)"() -> ("Value"=w330:dbl)  [unwired: 2 in, 2 out]
              n149 = property on="Scanrate (pixels/s)" class="Ring (strict)"() -> ("Value"=w335:i32)  [unwired: 2 in, 2 out]
              n150 = Add(x=w332, y=w349) -> (x+y=w336:dbl)
              n151 = property on="Z-Stacking" class="Bool (strict)"() -> ("Value"=w346:bool)  [unwired: 2 in, 2 out]
              n152 = Subtract(x=w331, y=w330) -> (x-y=w329:dbl)
              n153 = Multiply(x=w332, y=w336) -> (x*y=w350:dbl)
              n154 = Add(x=w350, y=w349) -> (x+y=w348:dbl)
              n155 = Divide(x=w336, y=w335) -> (x/y=w334:dbl)
              n156 = Divide(x=w329, y="Schritte") -> (x/y=w328:dbl)
              n157 = Divide(x=w348, y=w335) -> (x/y=w345:dbl)
              n158 = Select(t="Schritte", s=w346, f=1.0) -> (s? t:f=w344:dbl)
              n159 = property on="Schrittweite" class="DigNum (strict)"("Value"=w328) -> ()  [unwired: 2 in, 2 out]
              n160 = Multiply(x=w344, y=w345) -> (x*y=w338:dbl)
              n161 = Quotient & Remainder(x=w338, y=60.0) -> (x-y*floor(x/y)=w325:dbl, floor(x/y)=w342:dbl)
              n162 = Divide(x=w325, y=100.0) -> (x/y=w326:dbl)
              n163 = Add(x=w326, y=w342) -> (x+y=w340:dbl)
              n164 = Number To Fractional String(number=w340, precision (6)=i16 2) -> (F-format string=→"Duration (m.s)":string)  [unwired: 2 in]
            }
            event "Fire": Value Change {
              n165 = event-data() -> ()  [unwired: 1 in, 6 out]
              n166 = property on="Magnification" class="DigNum (strict)"() -> ("Value"=w376:dbl)  [unwired: 2 in, 2 out]
              n167 = property on="Image" class="IntGraph (strict)"("Active Cursor"=u32 2) -> ("Cursor.Cursor Position:Cursor X"=w362:dbl, "Cursor.Cursor Position:Cursor Y"=w361:dbl)  [unwired: 2 in, 2 out]
              n168 = property on="Minimum" class="Slide (strict)"() -> ("Value"=w360:dbl)  [unwired: 2 in, 2 out]
              n169 = Multiply(x=w362, y=2.1342 ("x")) -> (x*y=w393:dbl)
              n170 = Divide(x=w360, y=20.0) -> (x/y=w356:dbl)
              n171 = Divide(x=w361, y=w409) -> (x/y=w354:dbl)
              n172 = Divide(x=w393, y=w409) -> (x/y=w355:dbl)
              n173 = Build Array(w354, w355, w356) -> (w395:dbl[])
              n174 = call "go_to_point.vi"("error in"=w358, "data"=w395) -> ("error out"=w391:errorcluster)
              n175 = call-poly <vilib>:"DAQmx Create Virtual Channel.vi"("frequency"="Pulse repetition rate", "counter"=tag "Dev1/ctr0", "error in"=w391) -> ("task out"=w404:refnum<k21>, "error out"=w403:errorcluster)  [unwired: 11 in]
              n176 = call-poly <vilib>:"DAQmx Timing.vi"("task/channels in"=w404, "samples per channel"="Number of shots", "error in"=w403) -> ("task out"=w402:refnum<k21>, "error out"=w401:errorcluster)  [unwired: 11 in]
              n177 = call <vilib>:"DAQmx Start Task.vi"("task/channels in"=w402, "error in"=w401) -> ("task out"=w400:refnum<k21>, "error out"=w399:errorcluster)  [unwired: 12 in]
              n178 = while {
                tunnel: w400 -> [w418]
                tunnel: w399 -> [w417]
                tunnel: [w416] -> w398
                tunnel: [w414] -> w397
                stop <- w410 stop-if-true
                n179 = call <vilib>:"DAQmx Is Task Done.vi"("task/channels in"=w418, "error in"=w417) -> ("task out"=w416:refnum<k21>, "task done?"=w412:bool, "error out"=w414:errorcluster)  [unwired: 11 in]
                n180 = Not(x="Fire") -> (.not. x?=w411:bool)
                n181 = Unbundle By Name(w414) -> ("status"=w413:bool)
                n182 = Compound Arithmetic op=OR(w413, w412, w411) -> (w410:bool)
              }
              n183 = Format Into String(format string="z-Position: %f\nPosition: %f;%f\nHWP: %f\nNumber of shots: %d\nRepetition rate: %f\nPower [mA]: %f\nPower (sync) [mW]: %f\nPower (nosync) [mW]: %f\nPulse width [fs]: %f\nNA: %f\nMagnification: %f", w360, w362, w361, "HWP", "Number of shots", "Pulse repetition rate", "Power mA", "Power mW sync", "Power mW nosync", "Pulse width fs", "NA", w376) -> (resulting string=w366:string)  [unwired: 2 in, 1 out]
              n184 = property on="Image" class="IntGraph (strict)"() -> ("X Scale.Range:Minimum"=w389:dbl, "Y Scale.Range:Minimum"=w388:dbl)  [unwired: 2 in, 2 out]
              n185 = Get Date/Time In Seconds() -> (seconds since 1Jan1904=w372:timestamp)
              n186 = property on="File identifier" class="Str"() -> ("Value"=w371:string)  [unwired: 2 in, 2 out]
              n187 = Multiply(x=w389, y=2.1342 ("x")) -> (x*y=w387:dbl)
              n188 = call <vilib>:"DAQmx Clear Task.vi"("task in"=w398, "error in"=w397) -> ("error out"=w364:errorcluster)  [unwired: 13 in]
              n189 = Format Date/Time String(time format string (%c)="%Y%m\\%Y%m%d\\", seconds (now)=w372) -> (date/time string=w373:string)  [unwired: 1 in]
              n190 = Divide(x=w388, y=w409) -> (x/y=w353:dbl)
              n191 = Divide(x=w387, y=w409) -> (x/y=w352:dbl)
              n192 = Concatenate Strings("Y:\\Data\\" ("string"), w373, w371, w359, "_fire.log" ("string")) -> (w367:string)
              n193 = String To Path(string=w367) -> (path=w369:path)
              n194 = property on="Fire" class="Bool (strict)"(error in=w364, "Value"=FALSE ("Fire")) -> (error out=w363:errorcluster)  [unwired: 1 in, 1 out]
              n195 = Build Array(w353, w352, w356) -> (w390:dbl[])
              n196 = call <vilib>:"Write Characters To File.vi"("append to file? (new file:F)"=TRUE, "character string"=w366, "file path (dialog if empty)"=w369) -> ()  [unwired: 2 in, 1 out]
              n197 = call "go_to_point.vi"("error in"=w363, "data"=w390) -> ("error out"=w357:errorcluster)
            }
            event "Bild speichern ...": Value Change {
              # "Der Benutzer will das Bild speichern. Der Dateiname wird zusammengestellt\naus der Zeit des Scans und dem File identifier. Die Datums-Ordner werden\nbei Bedarf automatisch erstellt. (Innerhalb des Sub-vis)"
              n198 = event-data() -> ()  [unwired: 1 in, 6 out]
              n199 = property on="Image" class="IntGraph (strict)"() -> ("Value"=w423:dbl[][])  [unwired: 2 in, 2 out]
              n200 = call "save_to_disk.vi"("character string"=w426, "Array"=w423, "File identifier"="File identifier") -> ("path"=→"path":path)
              n201 = property on="Bild speichern ..." class="Bool (strict)"("Value"=FALSE ("Bild speichern ...")) -> ()  [unwired: 2 in, 2 out]
            }
            event Timeout {
              # "Die Photodiode für die Mira-Power wird ausgelesen."
              n202 = event-data() -> ()  [unwired: 1 in, 3 out]
              n203 = call-poly <vilib>:"DAQmx Read.vi"("task/channels in"=w451, "error in"=w450) -> ("data"=w449:dbl[], "error out"=w446:errorcluster)  [unwired: 11 in, 1 out]
              n204 = call "sr510_poll.vi"("error in"=w446) -> ("error out"=w430:errorcluster, "Phase"=w435:string, "Sensitivity [mV]"=w436:string, "Locked"=w441:bool)  [unwired: 3 in, 1 out]
              n205 = call-poly <vilib>:"Mean.vi"("X"=w449) -> ("mean"=w447:dbl)  [unwired: 1 out]
              n206 = Unbundle By Name(w430) -> ("status"=w440:bool)
              n207 = Multiply(x=-1225.0, y=w447) -> (x*y=w439:dbl)
              n208 = Not(x=w440) -> (.not. x?=w442:bool)
              n209 = And(x=w441, y=w442) -> (x .and. y?=w437:bool)
              "Lock-in" <- w437
              n210 = Select(t=0.415, s=w437, f=1.0) -> (s? t:f=w445:dbl)
              n211 = Divide(x=w439, y=w445) -> (x/y=→"Mira Power (mW)":dbl)
              n212 = case shown="True" w437 {
                selector: w437 -> [w453 w456]
                tunnel: w436 -> [_ w455]
                tunnel: w435 -> [_ w454]
                frame False {
                  n213 = property on="Phase" class="Str"("Visible"=w453) -> ()  [unwired: 2 in, 2 out]
                  n214 = property on="Sensitivity" class="Str"("Visible"=w453) -> ()  [unwired: 2 in, 2 out]
                }
                frame True {
                  n215 = property on="Phase" class="Str"("Visible"=w456) -> ()  [unwired: 2 in, 2 out]
                  n216 = property on="Sensitivity" class="Str"("Visible"=w456) -> ()  [unwired: 2 in, 2 out]
                  "Sensitivity" <- w455
                  "Phase" <- w454
                }
              }
            }
            event "Swap Memory": Mouse Up {
              n217 = event-data() -> ()  [unwired: 1 in, 8 out]
              n218 = property on="Memory" class="IntGraph (strict)"(error in=w458) -> (error out=w463:errorcluster, "Value"=w467:dbl[][])  [unwired: 1 in, 1 out]
              n219 = property on="Image" class="IntGraph (strict)"(error in=w463) -> (error out=w462:errorcluster, "Value"=→"Memory":dbl[][])  [unwired: 1 in, 1 out]
              n220 = property on="Image" class="IntGraph (strict)"(error in=w462, "Value"=w467) -> (error out=w457:errorcluster)  [unwired: 1 in, 1 out]
              n221 = property on="Swap Memory" class="Bool (strict)"("Value"=FALSE ("Swap Memory")) -> ()  [unwired: 2 in, 2 out]
            }
            event "Minimum", "Maximum", "Schrittweite": Value Change {
              n222 = event-data() -> ()  [unwired: 1 in, 6 out]
              n223 = property on="Schrittweite" class="DigNum (strict)"() -> ("Value"=w479:dbl)  [unwired: 2 in, 2 out]
              n224 = In Range and Coerce(upper limit="Maximum", x="Minimum", lower limit=-100.0) -> (coerced(x)=w476:dbl)  [unwired: 1 out]
              n225 = In Range and Coerce(upper limit=100.0, x="Maximum", lower limit="Minimum") -> (coerced(x)=w477:dbl)  [unwired: 1 out]
              n226 = Subtract(x="Maximum", y="Minimum") -> (x-y=w480:dbl)
              n227 = Divide(x=w480, y=w479) -> (x/y=w478:dbl)
              n228 = Round Toward -Infinity(1:w478) -> (0:w470:dbl)
              n229 = property on="Schritte" class="DigNum (strict)"("Value"=w470) -> ()  [unwired: 2 in, 2 out]
              n230 = property on="Minimum val" class="DigNum (strict)"("Value"=w476) -> ()  [unwired: 2 in, 2 out]
              n231 = property on="Minimum" class="Slide (strict)"("Value"=w476, "Data Range:Maximum"="Maximum") -> ()  [unwired: 2 in, 2 out]
              n232 = property on="Maximum val" class="DigNum (strict)"("Value"=w477) -> ()  [unwired: 2 in, 2 out]
              n233 = property on="Maximum" class="Slide (strict)"("Value"=w477, "Data Range:Minimum"="Minimum") -> ()  [unwired: 2 in, 2 out]
            }
            event "Minimum val", "Maximum val": Value Change {
              n234 = event-data() -> ()  [unwired: 1 in, 6 out]
              n235 = In Range and Coerce(upper limit="Maximum val", x="Minimum val", lower limit=-100.0) -> (coerced(x)=w493:dbl)  [unwired: 1 out]
              n236 = In Range and Coerce(upper limit=100.0, x="Maximum val", lower limit="Minimum val") -> (coerced(x)=w491:dbl)  [unwired: 1 out]
              n237 = property on="Schrittweite" class="DigNum (strict)"() -> ("Value"=w497:dbl)  [unwired: 2 in, 2 out]
              n238 = Subtract(x=w493, y=w491) -> (x-y=w498:dbl)
              n239 = Divide(x=w498, y=w497) -> (x/y=w496:dbl)
              n240 = Round Toward -Infinity(1:w496) -> (0:w486:dbl)
              n241 = property on="Schritte" class="DigNum (strict)"("Value"=w486) -> ()  [unwired: 2 in, 2 out]
              n242 = property on="Minimum val" class="DigNum (strict)"("Value"=w493) -> ()  [unwired: 2 in, 2 out]
              n243 = property on="Minimum" class="Slide (strict)"("Value"=w493, "Data Range:Maximum"="Maximum val") -> ()  [unwired: 2 in, 2 out]
              n244 = property on="Maximum val" class="DigNum (strict)"("Value"=w491) -> ()  [unwired: 2 in, 2 out]
              n245 = property on="Maximum" class="Slide (strict)"("Value"=w491, "Data Range:Minimum"="Minimum val") -> ()  [unwired: 2 in, 2 out]
            }
            event "Go to white point": Value Change {
              w516 = FALSE ("Go to black point")
              n246 = event-data() -> ()  [unwired: 1 in, 6 out]
              n247 = property on="Image" class="IntGraph (strict)"(error in=w505, "Active Cursor"=u32 2) -> (error out=w512:errorcluster, "Cursor.Cursor Position:Cursor X"=w511:dbl, "Cursor.Cursor Position:Cursor Y"=w519:dbl)  [unwired: 1 in, 1 out]
              n248 = property on="Minimum" class="Slide (strict)"() -> ("Value"=w507:dbl)  [unwired: 2 in, 2 out]
              n249 = Multiply(x=2.1342, y=w511) -> (x*y=w518:dbl)
              n250 = Divide(x=w507, y=20.0) -> (x/y=w503:dbl)
              n251 = Divide(x=w519, y=w521) -> (x/y=w501:dbl)
              n252 = Divide(x=w518, y=w521) -> (x/y=w502:dbl)
              n253 = Build Array(w501, w502, w503) -> (w522:dbl[])
              n254 = call "go_to_point.vi"("error in"=w512, "data"=w522) -> ("error out"=w514:errorcluster)
              n255 = property on="Go to white point" class="Bool (strict)"(error in=w514, "Value"=w516) -> (error out=w513:errorcluster)  [unwired: 1 in, 1 out]
              n256 = property on="Go home" class="Bool (strict)"(error in=w513, "Value"=w516, "Disabled"=u8 0) -> (error out=w504:errorcluster)  [unwired: 1 in, 1 out]
            }
            event "Go home": Value Change {
              n257 = event-data() -> ()  [unwired: 1 in, 6 out]
              n258 = Boolean To (0,1)(Boolean="Go home") -> (0, 1=w534:i16)
              n259 = property on="Go home" class="Bool (strict)"("Disabled"=w534) -> ()  [unwired: 2 in, 2 out]
              n260 = Initialize Array(u32 0 ("Active Cursor"), 3 ("dimension size")) -> (w526:u32[])
              n261 = call "go_to_point.vi"("error in"=w528, "data"=w526) -> ("error out"=w527:errorcluster)
            }
            event "black point": Value Change {
              n262 = event-data() -> ()  [unwired: 1 in, 6 out]
              n263 = property on="Image" class="IntGraph (strict)"("Active Cursor"=u32 2) -> ("Cursor.Cursor Position:Cursor X"=w562:dbl, "Cursor.Cursor Position:Cursor Y"=w561:dbl)  [unwired: 2 in, 2 out]
              n264 = property on="Grösse manuell" class="DigNum (strict)"() -> ("Value"=w542:dbl)  [unwired: 2 in, 2 out]
              n265 = Divide(x=w562, y=w543) -> (x/y=w559:dbl)
              n266 = Divide(x=w561, y=w543) -> (x/y=w560:dbl)
              n267 = Divide(x=w542, y=w543) -> (x/y=w541:dbl)
              n268 = Divide(x=w541, y=2.0) -> (x/y=w572:dbl)
              n269 = flat-sequence {
                frame #0 {
                  n270 = Wait (ms)(milliseconds to wait=u32 250) -> ()  [unwired: 1 out]
                }
                frame #1 {
                  n271 = Not(x="black point") -> (.not. x?=w575:bool)
                  n272 = property on="black point" class="Bool (strict)"("Value"=w575) -> ()  [unwired: 2 in, 2 out]
                }
              }
              n273 = Subtract(x=6.0, y=w541) -> (x-y=w567:dbl)
              n274 = Divide(x=w567, y=2.0) -> (x/y=w564:dbl)
              n275 = Multiply(x=1.0, y=w564) -> (x*y=w554:dbl)
              n276 = Negate(x=w554) -> (-x=w565:dbl)
              n277 = In Range and Coerce(upper limit=w554, x=w560, lower limit=w565) -> (coerced(x)=w558:dbl)  [unwired: 1 out]
              n278 = Add(x=w572, y=w558) -> (x+y=w549:dbl)
              n279 = Subtract(x=w558, y=w572) -> (x-y=w551:dbl)
              n280 = In Range and Coerce(upper limit=w554, x=w559, lower limit=w565) -> (coerced(x)=w557:dbl)  [unwired: 1 out]
              n281 = Subtract(x=w557, y=w572) -> (x-y=w550:dbl)
              n282 = Add(x=w557, y=w572) -> (x+y=w548:dbl)
              n283 = Multiply(x=w543, y=w557) -> (x*y=w556:dbl)
              n284 = Multiply(x=w558, y=w543) -> (x*y=w555:dbl)
              n285 = property on="x-Offset" class="DigNum (strict)"("Value"=w556) -> ()  [unwired: 2 in, 2 out]
              n286 = property on="y-Offset" class="DigNum (strict)"("Value"=w555) -> ()  [unwired: 2 in, 2 out]
              n287 = Multiply(x=w543, y=w548) -> (x*y=w547:dbl)
              n288 = Multiply(x=w543, y=w549) -> (x*y=w546:dbl)
              n289 = Multiply(x=w543, y=w550) -> (x*y=w545:dbl)
              n290 = Multiply(x=w543, y=w551) -> (x*y=w544:dbl)
              n291 = Multiply(x=w543, y=w554) -> (x*y=w553:dbl)
              n292 = Negate(x=w553) -> (-x=w552:dbl)
              n293 = property on="Image" class="IntGraph (strict)"("Active Cursor"=u32 0, "Cursor.Cursor Position:Cursor X"=w547, "Cursor.Cursor Position:Cursor Y"=w546, "Active Cursor"=u32 1, "Cursor.Cursor Position:Cursor X"=w545, "Cursor.Cursor Position:Cursor Y"=w544) -> ()  [unwired: 2 in, 2 out]
              n294 = property on="x-Offset" class="DigNum (strict)"("Data Range:Minimum"=w552, "Data Range:Maximum"=w553) -> ()  [unwired: 2 in, 2 out]
              n295 = property on="y-Offset" class="DigNum (strict)"("Data Range:Minimum"=w552, "Data Range:Maximum"=w553) -> ()  [unwired: 2 in, 2 out]
            }
            event "Piezo Stage": Value Change {
              n296 = event-data() -> ("NewVal"=w584:bool)  [unwired: 1 in, 5 out]
              n297 = Not(x=w584) -> (.not. x?=w577:bool)
              n298 = property on="Magnification" class="DigNum (strict)"() -> ("Value"=w582:dbl)  [unwired: 2 in, 2 out]
              n299 = Divide(x=13440.0, y=w582) -> (x/y=w588:dbl)
              n300 = call-poly <vilib>:"DAQmx Write.vi"("task/channels in"=w593, "data"=w584, "error in"=w594) -> ("error out"=w578:errorcluster)  [unwired: 10 in, 2 out]
              n301 = Select(t=w588, s=w577, f=20.0) -> (s? t:f=w579:dbl)
              n302 = Multiply(x=w579, y=w583) -> (x*y=w586:dbl[])
              n303 = for {
                tunnel: w586 -> [w596] mode=indexing
                tunnel: [w600] -> w585 mode=indexing
                tunnel: w583 -> [w599] mode=indexing
                n304 = Format Into String(format string="%dx%d \\B5m", w596, w596) -> (resulting string=w597:string)  [unwired: 2 in, 1 out]
                n305 = Bundle(w597, w599) -> (w600:cluster{string, dbl})  [unwired: 1 in]
              }
              n306 = property on="Grösse" class="Ring (strict)"("Strings And Values []"=w585) -> ("Value"=w581:dbl)  [unwired: 2 in, 2 out]
              n307 = Multiply(x=w579, y=w581) -> (x*y=w580:dbl)
              n308 = property on="Grösse manuell" class="DigNum (strict)"("Value"=w580) -> ()  [unwired: 2 in, 2 out]
            }
          }
        }
        n309 = property on="x-Offset" class="DigNum (strict)"(error in=w104) -> (error out=w103:errorcluster, "Value"=w112:dbl)  [unwired: 1 in, 1 out]
        n310 = property on="y-Offset" class="DigNum (strict)"(error in=w103) -> (error out=w106:errorcluster, "Value"=w113:dbl)  [unwired: 1 in, 1 out]
        n311 = property on="Grösse manuell" class="DigNum (strict)"(error in=w106) -> (error out=w105:errorcluster, "Value"=w111:dbl)  [unwired: 1 in, 1 out]
        n312 = Multiply(x=w113, y=w110) -> (x*y=w129:dbl)
        n313 = Multiply(x=w112, y=w110) -> (x*y=w127:dbl)
        n314 = Scale By Power Of 2(n=i16 1, x=w110) -> (x*2^n=w108:dbl)
        n315 = Divide(x=w111, y=w108) -> (x/y=w109:dbl)
        n316 = Format Into String(format string="x-offset: %f\ny-offset: %f\nAmplitude: %f\nAufloesung: %f\n", w127, w129, w111, w139) -> (resulting string=w118:string)  [unwired: 2 in, 1 out]
        n317 = property on="Mira Power (mW)" class="DigNum (strict)"() -> ("Value"=w125:dbl)  [unwired: 2 in, 2 out]
        n318 = property on="NA" class="DigNum (strict)"() -> ("Value"=w123:dbl)  [unwired: 2 in, 2 out]
        n319 = property on="Lock-in" class="Bool (strict)"() -> ("Value"=w100:bool)  [unwired: 2 in, 2 out]
        n320 = case shown="True" w100 {
          tunnel: ["" w604] -> w116
          tunnel: [w601 w609] -> w102
          tunnel: w105 -> [w601 w603]
          frame False {
          }
          frame True {
            n321 = call "sr510_poll.vi"("error in"=w603) -> ("error out"=w609:errorcluster, "Time constant [s]"=w605:string, "Phase"=w606:string, "Sensitivity [mV]"=w607:string)  [unwired: 3 in, 1 out]
            n322 = Format Into String(format string="Sensitivity [mV]: %s\nPhase: %s\nTime constant [s]: %s\n", w607, w606, w605) -> (resulting string=w604:string)  [unwired: 2 in, 1 out]
          }
        }
        n323 = property on="Scanrate (pixels/s)" class="Ring (strict)"() -> ("Value"=w114:i32)  [unwired: 2 in, 2 out]
        n324 = property on="Minimum" class="Slide (strict)"() -> ("Value"=w99:dbl)  [unwired: 2 in, 2 out]
        n325 = property on="Maximum" class="Slide (strict)"() -> ("Value"=w98:dbl)  [unwired: 2 in, 2 out]
        n326 = property on="Schritte" class="DigNum (strict)"() -> ("Value"=w96:dbl)  [unwired: 2 in, 2 out]
        n327 = Format Into String(format string="Mira-Power [mW]: %f\nred obj magn: %f\nred NA: %f\ngreen obj magn: %f\ngreen NA: %f\nred PMT-gain: %f\ngreen PMT-gain: %f\nLock-in: %d\nScanrate (pixels/s): %d\nz-Minimum: %f\nz-Maximum: %f\nstep-value: %f\nnumber of steps: %d\n", initial string=w118, w125, "Magn", w123, "Magn", "NA 2", "red PMT-gain", "green PMT-gain", w100, w114, w99, w98, "Schrittweite", w96) -> (resulting string=w117:string)  [unwired: 1 in, 1 out]
        n328 = Concatenate Strings(w117, w116) -> (w101:string)
      }
      frame #1 {
      }
      frame #2 {
        # "Hier werden die benötigten Wellenformen für den Analog-Ausgang des USB-6259 er-\nmittelt. Sie hängen ab von der Grösse, der Scanrate und der Samplerate. Die Wellen-\nformen werden berechnet.\nAusserdem werden die Skalen der Graphen an die Grösse angepasst, und die letzten\nWerte für das .info-File ausgegeben."
        n329 = Decrement(x=w657) -> (x-1=w665:dbl)
        n330 = property on="Piezo Stage" class="Bool (strict)"() -> ("Value"=w620:bool)  [unwired: 2 in, 2 out]
        n331 = Reciprocal(x=w665) -> (1/x=w664:dbl)
        n332 = Multiply(x=w664, y=2.0) -> (x*y=w662:dbl)
        n333 = Not(x=w620) -> (.not. x?=w619:bool)
        n334 = Multiply(x=w658, y=w662) -> (x*y=w638:dbl)
        n335 = Subtract(x=w626, y=w658) -> (x-y=w624:dbl)
        n336 = Subtract(x=w624, y=w638) -> (x-y=w640:dbl)
        n337 = for {
          N: w657 -> [_]
          tunnel: w638 -> [w691]
          tunnel: [w689] -> w660 mode=indexing
          shift-right: [w689] -> w661
          shift-left: w640 -> [w690]
          n338 = Add(x=w691, y=w690) -> (x+y=w689:dbl)
        }
        n339 = Select(t=u8 5, s=w619, f=u8 2) -> (s? t:f=w631:u8)
        n340 = Select(t=2.1342, s=w619, f=1.0) -> (s? t:f=w628:dbl)
        n341 = Divide(x=w657, y=w631) -> (x/y=w666:dbl)
        n342 = Multiply(x=w638, y=w631) -> (x*y=w636:dbl)
        n343 = Round Toward -Infinity(1:w666) -> (0:w645:dbl)
        n344 = Subtract(x=w627, y=w658) -> (x-y=w625:dbl)
        n345 = for {
          N: w645 -> [_]
          shift-right: [w686] -> _
          shift-left: w661 -> [w688]
          tunnel: w636 -> [w687]
          tunnel: [w686] -> w659 mode=indexing
          n346 = Subtract(x=w688, y=w687) -> (x-y=w686:dbl)
        }
        n347 = Add(x=w627, y=w658) -> (x+y=w672:dbl)
        n348 = Add(x=w626, y=w658) -> (x+y=w671:dbl)
        n349 = Multiply(x=2.0, y=w658) -> (x*y=w675:dbl)
        n350 = Divide(x=w675, y=w657) -> (x/y=w670:dbl)
        n351 = Multiply(x=w638, y=w628) -> (x*y=w637:dbl)
        n352 = Multiply(x=w628, y=w625) -> (x*y=w634:dbl)
        n353 = Build Array (concatenate)(w660, w659) -> (w652:dbl[])
        n354 = Subtract(x=w634, y=w637) -> (x-y=w639:dbl)
        n355 = Multiply(x=w667, y=w670) -> (x*y=w644:dbl)
        n356 = Multiply(x=w667, y=w672) -> (x*y=w642:dbl)
        n357 = Multiply(x=w667, y=w671) -> (x*y=w641:dbl)
        n358 = Negate(x=w644) -> (-x=w643:dbl)
        n359 = Multiply(x=w636, y=w628) -> (x*y=w635:dbl)
        n360 = Add(x=w657, y=w645) -> (x+y=w646:dbl)
        n361 = for {
          N: w657 -> [_]
          tunnel: w637 -> [w685]
          shift-right: [w682] -> w653
          shift-left: w639 -> [w684]
          tunnel: w652 -> [w683]
          tunnel: [w683] -> w656 mode=indexing
          tunnel: [w681] -> w654 mode=indexing
          tunnel: w646 -> [w680]
          n362 = Add(x=w685, y=w684) -> (x+y=w682:dbl)
          n363 = Initialize Array(w682, w680) -> (w681:dbl[])
        }
        n364 = Multiply(x=w657, y=w646) -> (x*y=w655:dbl)
        n365 = property on="Image" class="IntGraph (strict)"("X Scale.Offset and Multiplier:Multiplier"=w643, "X Scale.Offset and Multiplier:Offset"=w642, "Y Scale.Offset and Multiplier:Multiplier"=w643, "Y Scale.Offset and Multiplier:Offset"=w641) -> ()  [unwired: 2 in, 2 out]
        n366 = Reshape Array(w656, w655) -> (w651:dbl[])
        n367 = Reshape Array(w654, w655) -> (w648:dbl[])
        n368 = for {
          N: w645 -> [_]
          shift-right: [w677] -> _
          shift-left: w653 -> [w679]
          tunnel: w635 -> [w678]
          tunnel: [w677] -> w649 mode=indexing
          tunnel: w624 -> [w676]
          tunnel: [w676] -> w650 mode=indexing
          n369 = Subtract(x=w679, y=w678) -> (x-y=w677:dbl)
        }
        n370 = Build Array (concatenate)(w651, w650) -> (w623:dbl[])
        n371 = Build Array (concatenate)(w648, w649) -> (w622:dbl[])
        n372 = Build Array(w623, w622) -> (w647:dbl[][])
      }
      frame #3 {
        w734 = 10178 items=["Finite Samples"=10178, "Continuous Samples"=10123, "Hardware Timed Single Point"=12522] ("sample mode")
        w743 = 10106 items=["default"=-1, "RSE"=10083, "NRSE"=10078, "Differential"=10106, "Pseudodifferential"=12529] ("input terminal configuration")
        w737 = 10348 items=["Volts"=10348, "From Custom Scale"=10065] ("units")
        w763 = path "Y:/scan.log" ("path to log")
        # "Auflösung"
        # "Anzahl Pixel\npro Reihe"
        # "Die Aufträge des USB-6259 werden gelöscht.\nDie Cursor werden an den Rand des Graphen versetzt.\nFalls ein Z-Stacking läuft werden die Daten von EINEM Bild\nan ein File angehängt und das zugehörige .info-File geschrieben.\nAusserdem wird der \"Bild speichern\"-Knopf eingeblendet, falls\nkein Z-Stacking gelaufen ist. (\"Bild Speichern visibility\"=\"true\"\nvor dem ersten Frame.)"
        n373 = call-poly <vilib>:"DAQmx Create Virtual Channel.vi"("maximum value"=5.0, "minimum value"=-5.0, "physical channels"=tag "Dev1/ao2", "error in"=w753) -> ("task out"=w752:refnum<k21>, "error out"=w710:errorcluster)  [unwired: 10 in]
        n374 = Build Array(tag "Dev1/ai3" ("physical channels"), tag "Dev1/ai4" ("element")) -> (w735:tag[])
        n375 = call <vilib>:"DAQmx Flatten Channel String.vi"("names in"=w735, "error in"=w710) -> ("names out"=w750:string, "error out"=w747:errorcluster)  [unwired: 12 in]
        n376 = Build Array(tag "Dev1/ao0" ("physical channels"), tag "Dev1/ao1" ("physical channels")) -> (w739:tag[])
        n377 = call-poly <vilib>:"DAQmx Create Virtual Channel.vi"("maximum value"="maximum", "minimum value"="minimum", "input terminal configuration"=w743, "physical channels"=w750, "units"=w737, "error in"=w747) -> ("task out"=w714:refnum<k21>, "error out"=w709:errorcluster)  [unwired: 8 in]
        n378 = call <vilib>:"DAQmx Flatten Channel String.vi"("names in"=w739, "error in"=w709) -> ("names out"=w740:string, "error out"=w741:errorcluster)  [unwired: 12 in]
        n379 = call-poly <vilib>:"DAQmx Create Virtual Channel.vi"("maximum value"=3.0, "minimum value"=-3.0, "physical channels"=w740, "units"=w737, "error in"=w741) -> ("task out"=w717:refnum<k21>, "error out"=w708:errorcluster)  [unwired: 9 in]
        n380 = Divide(x=500000.0 ("rate"), y="Scanrate (pixels/s)") -> (x/y=w721:dbl)
        n381 = Round Toward -Infinity(1:w721) -> (0:w693:dbl)
        n382 = Multiply(x=w720, y=w693) -> (x*y=w729:dbl)
        n383 = Add(x=w720, y=w719) -> (x+y=w727:dbl)
        n384 = call-poly <vilib>:"DAQmx Timing.vi"("task/channels in"=w717, "sample mode"=w734, "samples per channel"=w727, "rate"="Scanrate (pixels/s)", "error in"=w708) -> ("task out"=w716:refnum<k21>, "error out"=w726:errorcluster)  [unwired: 9 in]
        n385 = Multiply(x=w693, y="Scanrate (pixels/s)") -> (x*y=w732:dbl)
        n386 = Max & Min(x=w729, y=25000000.0) -> (min(x,y)=w731:dbl)  [unwired: 1 out]
        n387 = call-poly <vilib>:"DAQmx Trigger.vi"("task/channels in"=w716, "source"=tag "/Dev1/ai/StartTrigger", "error in"=w726) -> ("task out"=w715:refnum<k21>, "error out"=w707:errorcluster)  [unwired: 11 in]
        n388 = call <vilib>:"DAQmx Configure Input Buffer.vi"("task/channels in"=w714, "buffer size (in samples per channel)"=w731, "error in"=w707) -> ("task out"=w713:refnum<k21>, "error out"=w730:errorcluster)  [unwired: 11 in]
        n389 = call-poly <vilib>:"DAQmx Timing.vi"("task/channels in"=w713, "sample mode"=w734, "samples per channel"=w729, "rate"=w732, "error in"=w730) -> ("task out"=w712:refnum<k21>, "error out"=w733:errorcluster)  [unwired: 9 in]
        n390 = property class="DAQmx Read"(reference=w712, error in=w733, "Read All Available Samples"=TRUE ("ReadAllAvailSamp")) -> (reference out=w711:refnum<k21>, error out=w706:errorcluster)
        n391 = Multiply(x="Buffer Size", y=w693) -> (x*y=w694:dbl)
        n392 = Bundle(w694, u32 2) -> (w724:cluster{dbl, u32})  [unwired: 1 in]
        n393 = call-poly <userlib>:"Circular Buffer.vi"("Buffer Size"=w724, "error in (no error)"=w706, "Operation"=Circular_Buffer_Operations."Initialize") -> ("error out"=w705:errorcluster)  [unwired: 5 in, 3 out]
        n394 = while {
          tunnel: w770 -> [w847]
          tunnel: w769 -> [w844]
          tunnel: w768 -> [w843]
          tunnel: [w811] -> w701
          tunnel: [w800] -> w767
          tunnel: [w841] -> w762
          tunnel: [w840] -> w761
          tunnel: [w813] -> w702
          tunnel: w719 -> [_]
          tunnel: w720 -> [_]
          tunnel: w757 -> [w835]
          shift-right: [w806] -> w700
          shift-left: w705 -> [w802]
          tunnel: w752 -> [w817]
          tunnel: [w816] -> w751
          tunnel: w711 -> [w804]
          tunnel: w715 -> [w805]
          tunnel: w696 -> [w795]
          tunnel: w695 -> [w794]
          tunnel: w694 -> [w792]
          tunnel: w693 -> [w791]
          stop <- w793 stop-if-true
          # "Buffer size"
          # "Die ermittelten Wellenformen für x und y werden zusammengeführt und auf zwei analoge Aus-\ngänge des USB-6259 geschrieben. Zudem wird das Auslesen initialisiert. Die Ausgänge (Wellen-\nformen) werden auf ein automatisch vom Gerät erzeugtes Startsignal des Einganges (Auslesen)\ngetriggert.\n\nDer Eingang wird im referenced single ended modus betrieben.\n\nDanach wird zuerst der Ausgang gestartet, der auf den Trigger wartet, der erfolgt, wenn das \nAuslesen gestartet wird. Der Ausgang erwartet 4*Auflösung^2 Samples zum Auslesen, mit einer\nSamplerate, die sich aus (lines per second)/(2*Auflösung)*(Anzahl Samples) ergibt. (I.e.\n(lines per second)/(number of lines)*(number of samples).)"
          # "Samples\npro Pixel"
          # "Die Daten werden ausgelesen. Sie folgen in einem 1D-Array, der entsprechend\nder Auflösung umgeformt wird. Da in einem Durchgang jeder Punkt viermal\naufgenommen wird (da zwei Dreiecks-Wellenformen benutzt werden), wird der\nArray in vier Bilder aufgeteilt und dargestellt."
          n395 = Divide(x="z-Position", y=20.0) -> (x/y=w828:dbl)
          n396 = call-poly <vilib>:"DAQmx Write.vi"("task/channels in"=w817, "auto start"=TRUE, "data"=w828, "error in"=w802) -> ("task out"=w826:refnum<k21>, "error out"=w825:errorcluster)  [unwired: 9 in, 1 out]
          n397 = call <vilib>:"DAQmx Wait Until Done.vi"("task/channels in"=w826, "error in"=w825) -> ("task out"=w816:refnum<k21>, "error out"=w815:errorcluster)  [unwired: 12 in]
          n398 = call-poly <vilib>:"DAQmx Write.vi"("task/channels in"=w805, "auto start"=FALSE, "data"=w835, "error in"=w815) -> ("task out"=w833:refnum<k21>, "error out"=w834:errorcluster)  [unwired: 9 in, 1 out]
          n399 = call <vilib>:"DAQmx Start Task.vi"("task/channels in"=w833, "error in"=w834) -> ("task out"=w814:refnum<k21>, "error out"=w838:errorcluster)  [unwired: 12 in]
          n400 = call <vilib>:"DAQmx Start Task.vi"("task/channels in"=w804, "error in"=w838) -> ("task out"=w846:refnum<k21>, "error out"=w839:errorcluster)  [unwired: 12 in]
          n401 = Decrement(x=w844) -> (x-1=w845:dbl)
          n402 = Subtract(x=w844, y=w843) -> (x-y=w842:dbl)
          n403 = Initialize Array(0.0 ("element"), w844, w844) -> (w832:dbl[][])
          n404 = while {
            tunnel: w791 -> [w901]
            shift-right: [w894] -> w840
            shift-left: w845 -> [w899]
            shift-right: [w883] -> w841
            shift-left: w845 -> [w898]
            tunnel: w847 -> [w897]
            tunnel: w845 -> [w896]
            shift-right: [w895] -> w796
            shift-left: w832 -> [w900]
            shift-right: [w893] -> w808
            shift-left: w839 -> [w904]
            tunnel: w842 -> [w892]
            tunnel: w792 -> [w885]
            shift-right: [w881] -> w789
            shift-left: w832 -> [w882]
            stop <- w889 stop-if-true
            # "x-counter"
            # "y-counter"
            n405 = call-poly <userlib>:"Circular Buffer.vi"("error in (no error)"=w904, "Operation"=Circular_Buffer_Operations."Get Backlog") -> ("error out"=w903:errorcluster, "Elements Remaining"=w886:i32)  [unwired: 6 in, 2 out]
            n406 = Divide(x=w886, y=w885) -> (x/y=→"Buffer":dbl)
            n407 = Greater Or Equal?(x=w886, y=w901) -> (x >= y?=w902:bool)
            n408 = case shown="True" w902 {
              tunnel: w903 -> [w907 w930]
              tunnel: w901 -> [_ w928]
              tunnel: w900 -> [w908 w926]
              tunnel: w899 -> [w910 w915]
              tunnel: w898 -> [w909 w924]
              tunnel: w897 -> [_ w923]
              tunnel: w896 -> [_ w922]
              tunnel: [w908 w921] -> w895
              tunnel: [w910 w920] -> w894
              tunnel: [w909 w919] -> w883
              tunnel: [w907 w912] -> w893
              tunnel: w892 -> [_ w917]
              tunnel: w882 -> [w906 w914]
              tunnel: [w906 w911] -> w881
              frame False {
              }
              frame True {
                n409 = Equal?(x=w917, y=w915) -> (x = y?=w918:bool)
                n410 = call-poly <userlib>:"Circular Buffer.vi"("error in (no error)"=w930, "Read Size"=w928, "Operation"=Circular_Buffer_Operations."Read (continuous)") -> ("error out"=w913:errorcluster, "Data Out"=w927:waveform(dbl)[])  [unwired: 5 in, 2 out]
                n411 = Greater Or Equal To 0?(x=w915) -> (x >= 0?=w916:bool)
                n412 = Decrement(x=w915) -> (x-1=w925:dbl)
                n413 = case shown="True" w916 {
                  tunnel: w927 -> [_ w947]
                  tunnel: w926 -> [w933 w944]
                  tunnel: w924 -> [_ w939]
                  tunnel: [w933 w942] -> w921
                  tunnel: w915 -> [_ w940]
                  tunnel: [w932 w941] -> w911
                  tunnel: w914 -> [w932 w943]
                  tunnel: w913 -> [w931 w946]
                  tunnel: [w931 w945] -> w912
                  frame False {
                  }
                  frame True {
                    n414 = call-poly <vilib>:"Basic Averaged DC-RMS.vi"("error in (no error)"=w946, "signals in"=w947) -> ("error out"=w945:errorcluster, "DC values"=w938:dbl[])  [unwired: 6 in, 2 out]
                    n415 = Index Array(array=w938, index #1=0 ("index"), index #2=1 ("index")) -> (element #1=w935:dbl, element #2=w934:dbl)
                    n416 = Replace Array Subset(array=w944, new element=w935, index (row)=w939, index (col)=w940) -> (w942:dbl[][])
                    n417 = Replace Array Subset(array=w943, new element=w934, index (row)=w939, index (col)=w940) -> (w941:dbl[][])
                  }
                }
                n418 = case shown="True" w918 {
                  tunnel: w924 -> [w949 w962]
                  tunnel: [w949 w961] -> w919
                  tunnel: w921 -> [_ w950]
                  tunnel: [w948 w964] -> w920
                  tunnel: w925 -> [w948 _]
                  tunnel: w922 -> [_ w964]
                  tunnel: w923 -> [_ w963]
                  tunnel: w911 -> [_ w951]
                  frame False {
                  }
                  frame True {
                    n419 = Multiply(x=w963, y=w962) -> (x*y=w954:dbl)
                    n420 = Decrement(x=w962) -> (x-1=w961:dbl)
                    n421 = Quotient & Remainder(x=w954, y=60.0) -> (x-y*floor(x/y)=w957:dbl, floor(x/y)=w959:dbl)
                    n422 = Divide(x=w957, y=100.0) -> (x/y=w958:dbl)
                    n423 = Add(x=w958, y=w959) -> (x+y=w955:dbl)
                    n424 = Number To Fractional String(number=w955, precision (6)=i16 2) -> (F-format string=w952:string)  [unwired: 2 in]
                    n425 = property on="Duration (m.s)" class="Str"("Value"=w952) -> ()  [unwired: 2 in, 2 out]
                    n426 = property on="Memory" class="IntGraph (strict)"("Value"=w951) -> ()  [unwired: 2 in, 2 out]
                    "Image" <- w950
                  }
                }
              }
            }
            n427 = property on="Scan" class="Bool (strict)"() -> ("Value"=w888:bool)  [unwired: 2 in, 2 out]
            n428 = Not(x=w888) -> (.not. x?=w887:bool)
            n429 = Unbundle By Name(w893) -> ("status"=w891:bool)
            n430 = Less Than 0?(x=w883) -> (x < 0?=w890:bool)
            n431 = Compound Arithmetic op=OR(w891, w890, w887) -> (w889:bool)
          }
          n432 = while {
            tunnel: w846 -> [w880]
            tunnel: [w869] -> w812
            shift-right: [w860] -> w810
            shift-left: w839 -> [w879]
            stop <- w873 stop-if-true
            w878 = -1.0 ("timeout")
            n433 = call-poly <vilib>:"DAQmx Read.vi"("task/channels in"=w880, "number of samples per channel"=w878, "timeout"=w878, "error in"=w879) -> ("task out"=w870:refnum<k21>, "data"=w877:waveform(dbl)[], "error out"=w875:errorcluster)  [unwired: 9 in]
            n434 = call-poly <userlib>:"Circular Buffer.vi"("error in (no error)"=w875, "Operation"=Circular_Buffer_Operations."Write", "Data In"=w877) -> ("error out"=w863:errorcluster)  [unwired: 5 in, 3 out]
            n435 = call <vilib>:"DAQmx Is Task Done.vi"("task/channels in"=w870, "error in"=w863) -> ("task out"=w864:refnum<k21>, "task done?"=w866:bool, "error out"=w862:errorcluster)  [unwired: 11 in]
            n436 = property class="DAQmx Read"(reference=w864, error in=w862) -> (reference out=w869:refnum<k21>, error out=w861:errorcluster, "AvailSampPerChan"=w868:u32)
            n437 = Equal To 0?(x=w868) -> (x = 0?=w867:bool)
            n438 = property on="Scan" class="Bool (strict)"(error in=w861) -> (error out=w860:errorcluster, "Value"=w874:bool)  [unwired: 1 in, 1 out]
            n439 = And(x=w867, y=w866) -> (x .and. y?=w865:bool)
            n440 = Unbundle By Name(w861) -> ("status"=w872:bool)
            n441 = Not(x=w874) -> (.not. x?=w871:bool)
            n442 = Compound Arithmetic op=OR(w872, w871, w865) -> (w873:bool)
          }
          n443 = property on="Z-Stacking" class="Bool (strict)"() -> ("Value"=w790:bool)  [unwired: 2 in, 2 out]
          n444 = call <vilib>:"DAQmx Stop Task.vi"("task/channels in"=w814, "error in"=w808) -> ("task out"=w813:refnum<k21>, "error out"=w807:errorcluster)  [unwired: 12 in]
          n445 = call <vilib>:"DAQmx Stop Task.vi"("task/channels in"=w812, "error in"=w810) -> ("task out"=w811:refnum<k21>, "error out"=w809:errorcluster)  [unwired: 12 in]
          n446 = Merge Errors(w807, w809) -> (w798:errorcluster)
          n447 = property on="Schritte" class="DigNum (strict)"(error in=w798) -> (error out=w822:errorcluster, "Value"=w824:dbl)  [unwired: 1 in, 1 out]
          n448 = Increment(x=w824) -> (x+1=w823:dbl)
          n449 = property on="Schritte" class="DigNum (strict)"(error in=w822, "Value"=w823) -> ()  [unwired: 1 in, 2 out]
          n450 = property on="Schrittweite" class="DigNum (strict)"(error in=w798) -> (error out=w819:errorcluster, "Value"=w831:dbl)  [unwired: 1 in, 1 out]
          n451 = property on="z-Position" class="DigNum (strict)"(error in=w798) -> (error out=w818:errorcluster, "Value"=w821:dbl)  [unwired: 1 in, 1 out]
          n452 = Add(x=w831, y=w821) -> (x+y=w829:dbl)
          n453 = property on="z-Position" class="DigNum (strict)"(error in=w819, "Value"=w829) -> ()  [unwired: 1 in, 2 out]
          n454 = property on="Maximum" class="Slide (strict)"(error in=w818) -> ("Value"=w830:dbl)  [unwired: 1 in, 2 out]
          n455 = Greater?(x=w829, y=w830) -> (0:w801:bool)
          n456 = Unbundle By Name(w798) -> ("status"=w797:bool)
          n457 = property on="Scan" class="Bool (strict)"(error in=w798) -> (error out=w806:errorcluster, "Value"=w800:bool)  [unwired: 1 in, 1 out]
          n458 = Not(x=w800) -> (.not. x?=w799:bool)
          n459 = Compound Arithmetic op=OR(w797, w799, w801) -> (w793:bool)
          n460 = case shown="True" w790 {
            tunnel: w794 -> [_ w852]
            tunnel: w795 -> [_ w849]
            tunnel: w796 -> [_ w857]
            tunnel: w793 -> [_ w856]
            tunnel: w789 -> [_ w853]
            frame False {
            }
            frame True {
              n461 = property on="File identifier" class="Str"() -> ("Value"=w850:string)  [unwired: 2 in, 2 out]
              n462 = Concatenate Strings(w850, w849) -> (w858:string)
              n463 = Concatenate Strings(w850, w849, "_trans" ("string")) -> (w851:string)
              n464 = Get Date/Time In Seconds() -> (seconds since 1Jan1904=w854:timestamp)
              n465 = call "append_to_disk.vi"("write info file?"=FALSE, "time stamp"=w854, "File identifier"=w851, "file info"=w852, "Data"=w853) -> ()  [unwired: 2 out]
              n466 = call "append_to_disk.vi"("write info file?"=w856, "time stamp"=w854, "File identifier"=w858, "file info"=w852, "Data"=w857) -> ("Path"=w859:path)  [unwired: 1 out]
              n467 = property on="path" class="Path"("Value"=w859) -> ()  [unwired: 2 in, 2 out]
            }
          }
        }
        n468 = call <vilib>:"DAQmx Clear Task.vi"("task in"=w751) -> ()  [unwired: 14 in, 1 out]
        n469 = Unbundle By Name(w700) -> ("status"=w766:bool, "code"=w765:i32, "source"=w764:string)
        n470 = case shown="True" w766 {
          tunnel: w765 -> [_ w968]
          tunnel: w764 -> [_ w967]
          tunnel: w763 -> [_ w972]
          tunnel: w761 -> [_ w965]
          tunnel: w762 -> [_ w966]
          frame False {
          }
          frame True {
            n471 = Get Date/Time In Seconds() -> (seconds since 1Jan1904=w969:timestamp)
            n472 = Format Into String(format string="%T: Error encountered: %d: %s. Scan will abort.\nLast sample aquired: %d,%d", w969, w968, w967, w966, w965) -> (resulting string=w970:string)  [unwired: 2 in, 1 out]
            n473 = call <vilib>:"Write Characters To File.vi"("append to file? (new file:F)"=TRUE, "character string"=w970, "file path (dialog if empty)"=w972) -> ()  [unwired: 2 in, 1 out]
          }
        }
        n474 = case shown="False" w767 {
          tunnel: w763 -> [w979 w984]
          tunnel: w762 -> [w977 _]
          tunnel: w761 -> [w976 _]
          frame False {
            n475 = Get Date/Time In Seconds() -> (seconds since 1Jan1904=w975:timestamp)
            n476 = Format Into String(format string="%T: Scan stopped. Sample %d,%d was the last one to be collected", w975, w977, w976) -> (resulting string=w974:string)  [unwired: 2 in, 1 out]
            n477 = call <vilib>:"Write Characters To File.vi"("append to file? (new file:F)"=TRUE, "character string"=w974, "file path (dialog if empty)"=w979) -> ()  [unwired: 2 in, 1 out]
          }
          frame True {
            n478 = Get Date/Time In Seconds() -> (seconds since 1Jan1904=w982:timestamp)
            n479 = Format Into String(format string="%T: Slice scan finished", w982) -> (resulting string=w981:string)  [unwired: 2 in, 1 out]
            n480 = call <vilib>:"Write Characters To File.vi"("append to file? (new file:F)"=TRUE, "character string"=w981, "file path (dialog if empty)"=w984) -> ()  [unwired: 2 in, 1 out]
          }
        }
        n481 = call <vilib>:"DAQmx Clear Task.vi"("task in"=w702, "error in"=w700) -> ("error out"=w788:errorcluster)  [unwired: 13 in]
        n482 = call <vilib>:"DAQmx Clear Task.vi"("task in"=w701, "error in"=w700) -> ("error out"=w787:errorcluster)  [unwired: 13 in]
        n483 = Merge Errors(w788, w787) -> (w760:errorcluster)
        n484 = property on="Image" class="IntGraph (strict)"(error in=w760) -> (error out=w759:errorcluster, "X Scale.Range:Minimum"=w775:dbl, "Y Scale.Range:Minimum"=w774:dbl, "X Scale.Range:Maximum"=w773:dbl, "Y Scale.Range:Maximum"=w772:dbl)  [unwired: 1 in, 1 out]
        n485 = Subtract(x=w772, y=w774) -> (x-y=w779:dbl)
        n486 = Unbundle By Name(w759) -> ("status"=w771:bool)
        "System" <- w771
        n487 = Divide(x=w779, y=2.0) -> (x/y=w777:dbl)
        n488 = Add(x=w777, y=w774) -> (x+y=w776:dbl)
        n489 = Subtract(x=w773, y=w775) -> (x-y=w783:dbl)
        n490 = Divide(x=w783, y=2.0) -> (x/y=w780:dbl)
        n491 = Add(x=w780, y=w775) -> (x+y=w782:dbl)
        n492 = property on="Image" class="IntGraph (strict)"(error in=w759, "Active Cursor"=u32 1, "Cursor.Cursor Position:Cursor X"=w775, "Cursor.Cursor Position:Cursor Y"=w774, "Active Cursor"=u32 0, "Cursor.Cursor Position:Cursor X"=w773, "Cursor.Cursor Position:Cursor Y"=w772, "Active Cursor"=u32 2, "Cursor.Cursor Position:Cursor X"=w782, "Cursor.Cursor Position:Cursor Y"=w776) -> (error out=w758:errorcluster)  [unwired: 1 in, 1 out]
        n493 = Not(x="Z-Stacking") -> (.not. x?=w697:bool)
      }
    }
  }
  n494 = call <vilib>:"Simple Error Handler.vi"("error in (no error)"=w40) -> ()  [unwired: 4 in, 5 out]
